vi "frontEnd.vi"() -> ()   [LabVIEW 2016]
uses:
  <userlib>/atmcd64d.llb/Error Code Enum typedef.ctl
  <userlib>/atmcd64d.llb/Shutter_mode typedef.ctl
  <userlib>/atmcd64d.llb/Shutter_type typedef.ctl
  <userlib>/atmcd64d.llb/FanMode_mode typedef.ctl
  <userlib>/atmcd64d.llb/ReadMode_mode typedef.ctl
  <userlib>/atmcd64d.llb/HSSpeed_type typedef.ctl
  <userlib>/atmcd64d.llb/AcquisitionMode_mode typedef.ctl
  <vilib>/Utility/miscctls.llb/LVStringsAndValuesArrayTypeDef_U16.ctl
  <vilib>/Utility/config.llb/Read Key (I32).vi
  <vilib>/Utility/config.llb/Read Key (Double).vi
  <vilib>/Instr/_visa.llb/VISA Configure Serial Port (Instr).vi
  <vilib>/Utility/config.llb/Read Key (String).vi
  <vilib>/Utility/config.llb/Write Key (String).vi
  <vilib>/Utility/config.llb/NI_LVConfig.lvlib
  lib/SSClassic_USBCamera_SDK.dll
panel:
  in  "String":string
  in  "Exposure Time:":dbl(slide) scale=1.0..100.0
  out "ET Labelµ":dbl format="%#_3g"
  out "new picture":picture
  in  "Red Gain":i32(slide)=20 scale=1.0..64.0
  in  "Green Gain":i32(slide)=16 scale=1.0..64.0
  in  "Blue Gain":i32(slide)=17 scale=1.0..64.0
  in  "Gain?":bool
  in  "gamma":i32=10 min=1 max=20
  in  "contrast":i32=50 min=0 max=100
  in  "bright":i32=50 min=0 max=100
  in  "sharp":i32 min=0 max=3
  out "ModuleNo:":string
  out "SerialNo:":string
  out "OK to run":bool
  in  "OM":bool
  out "relative seconds 2":dbl format="%_19f"
  out "relative seconds":dbl format="%_19f"
  out "Moving":bool
  in  "Go Origin":bool caption="Origin Return"
  in  "Set Origin":bool
  in  "Stage Position":string
  out "Cooler":bool
  out "Constructing data":u8(slide) scale=0.0..256.0
  in  "Go back after scan":bool=TRUE
  in  "Scan Step (um)":dbl
  in  "Step length (um)":dbl=100.0
  in  "go left Button":bool
  in  "go right Button":bool
  out "Y":dbl
  out "X":dbl
  in  "Scan again":bool
  in  "path":path
  in  "Bandwidth":dbl
  in  "Wavelength":i32(slide) scale=316.10943603515625..1105.4000244140625
  out "Waveform Graph":i32[](graph)
  out "Right Graph":i32[][](graph) caption="Object Image"
  out "recovering temperature":bool
  out "Left Graph":i32[][](graph) caption="On Sensor Image"
  out "Numeric 2":i32
  out "temp. status 2":T1
  out "model":string
  out "DLL error code from ini":u32
  in  "Save File":bool
  in  "Shut Down":bool
  in  "Scan Abort":bool
  out "Current \nScan Frame":dbl
  out "Total \nScan Frame":dbl
  in  "Scan Start":bool
  in  "Scan Length (mm)":dbl=25.0
  in  "Shutter Control":T2
  in  "Exposure Time (s)":sgl=0.01 step=0.001 format="%.4f"
  in  "Take shot":bool
  in  "VSS (s)":u16(ring) items=["0.300000", "0.500000", "0.900000", "1.700000", "3.300000"]
  in  "HSS (MHz)":i32(ring) items=["3", "1"]
  in  "Live View":bool
  out "Status":T1
  out "Temp":dbl
  in  "Set Temp.":dbl=20.0
  in  "Init File":path=path "C:/Users/Administrator/Desktop/micro.ini"
  # "Image Settigns"
  # "Stage Control"
  # "Scan"
  # "Save and Restart"
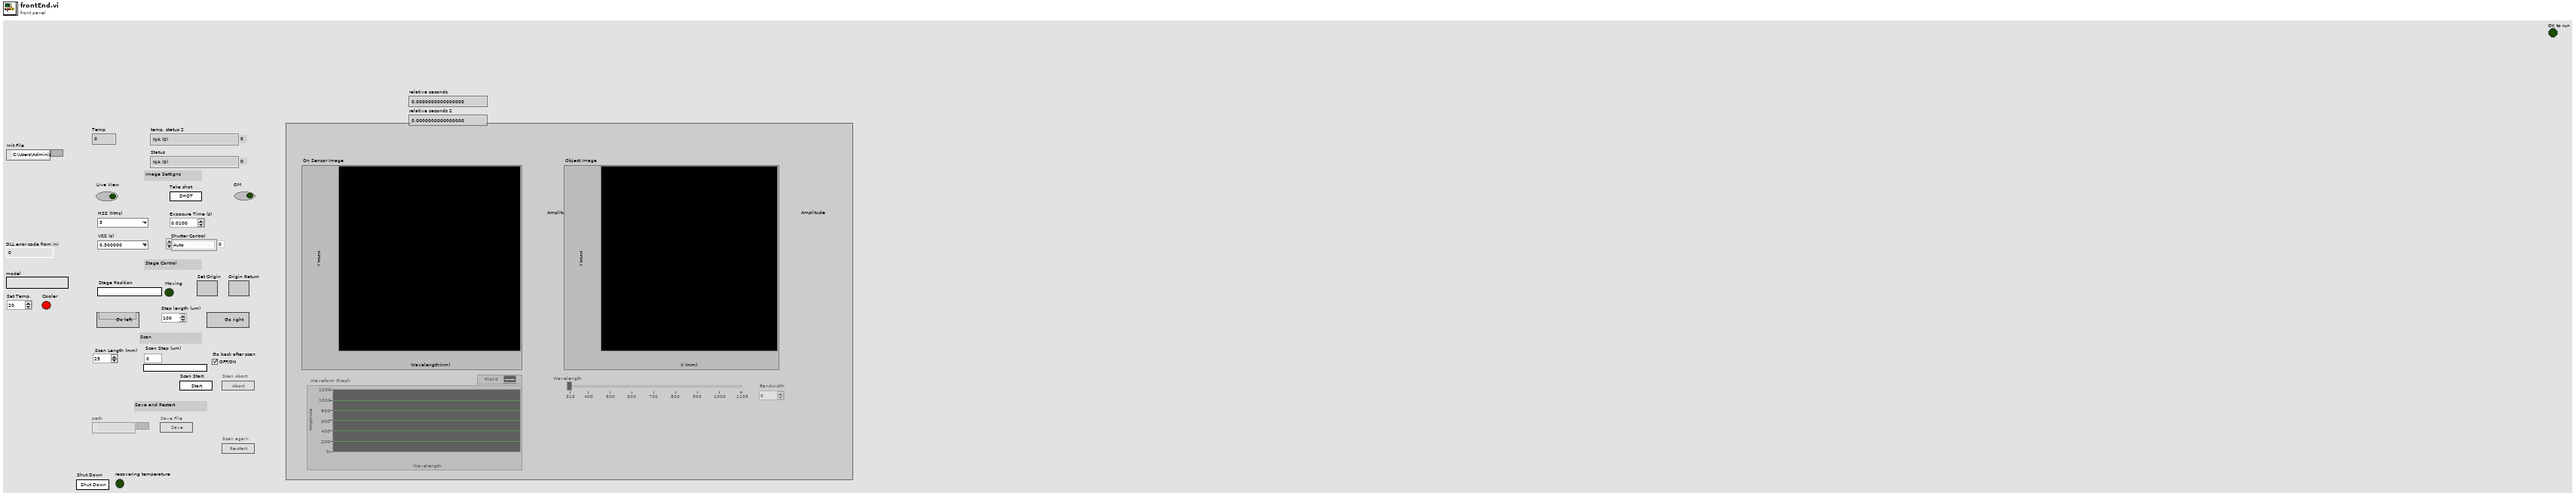
[diagram p1: front panel]
types:
  T1 = typedef "Error Code Enum typedef.ctl" = enum32{"N/A (0)", "DRV_ERROR_CODES", "DRV_SUCCESS", "DRV_VXDNOTINSTALLED", "DRV_ERROR_SCAN", "DRV_ERROR_CHECK_SUM", "DRV_ERROR_FILELOAD", "DRV_UNKNOWN_FUNC", "DRV_ERROR_VXD_INIT", "DRV_ERROR_ADDRESS", "DRV_ERROR_PAGELOCK", "DRV_ERROR_PAGEUNLOCK", "DRV_ERROR_BOARDTEST", "DRV_ERROR_ACK", "DRV_ERROR_UP_FIFO", "DRV_ERROR_PATTERN", "N/A (16)", "DRV_ACQUISITION_ERRORS", "DRV_ACQ_BUFFER", "DRV_ACQ_DOWNFIFO_FULL", "DRV_PROC_UNKONWN_INSTRUCTION", "DRV_ILLEGAL_OP_CODE", "DRV_KINETIC_TIME_NOT_MET", "DRV_ACCUM_TIME_NOT_MET", "DRV_NO_NEW_DATA", "N/A (25)", "DRV_SPOOLERROR", "N/A (27)", "N/A (28)", "N/A (29)", "N/A (30)", "N/A (31)", "N/A (32)", "DRV_TEMPERATURE_CODES", "DRV_TEMPERATURE_OFF", "DRV_TEMPERATURE_NOT_STABILIZED", "DRV_TEMPERATURE_STABILIZED", "DRV_TEMPERATURE_NOT_REACHED", "DRV_TEMPERATURE_OUT_RANGE", "DRV_TEMPERATURE_NOT_SUPPORTED", "DRV_TEMPERATURE_DRIFT", "N/A (41)", "N/A (42)", "N/A (43)", "N/A (44)", "N/A (45)", "N/A (46)", "N/A (47)", "N/A (48)", "DRV_GENERAL_ERRORS", "DRV_INVALID_AUX", "DRV_COF_NOTLOADED", "DRV_FPGAPROG", "DRV_FLEXERROR", "DRV_GPIBERROR", "N/A (55)", "N/A (56)", "N/A (57)", "N/A (58)", "N/A (59)", "N/A (60)", "N/A (61)", "N/A (62)", "N/A (63)", "DRV_DATATYPE", "DRV_DRIVER_ERRORS", "DRV_P1INVALID", "DRV_P2INVALID", "DRV_P3INVALID", "DRV_P4INVALID", "DRV_INIERROR", "DRV_COFERROR", "DRV_ACQUIRING", "DRV_IDLE", "DRV_TEMPCYCLE", "DRV_NOT_INITIALIZED", "DRV_P5INVALID", "DRV_P6INVALID", "DRV_INVALID_MODE", "DRV_INVALID_FILTER", "DRV_I2CERRORS", "DRV_I2CDEVNOTFOUND", "DRV_I2CTIMEOUT", "DRV_P7INVALID", "N/A (84)", "N/A (85)", "N/A (86)", "N/A (87)", "N/A (88)", "N/A (89)", "DRV_IOCERROR", "DRV_VRMVERSIONERROR"}
  T2 = typedef "Shutter_mode typedef.ctl" = enum16{"Auto", "Open", "Close", "N/A (3)", "Open FVB Series", "Open Any Series"}
  T3 = cluster{"Distance":i32, "Focal length":i32, "Y Range":i32}
  T4 = enum16{"open", "replace", "create", "open or create", "replace or create", "replace or create with confirmation"}
  T5 = typedef "FanMode_mode typedef.ctl" = enum16{"fan on full", "fan on low", "fan off"}
  T6 = typedef "Shutter_type typedef.ctl" = enum16{"TTL Low", "TTL High"}
  T7 = typedef "LVStringsAndValuesArrayTypeDef_U16.ctl" = cluster{"String":string, "Value":u16}[]
  T8 = typedef "AcquisitionMode_mode typedef.ctl" = enum16{"Reserved (0)", "Single Scan", "Accumulate", "Kinetics", "Fast Kinetics", "Run Till Abort", "Reserved (6)", "Reserved (7)", "Reserved (8)", "Time Delayed Integration"}
  T9 = typedef "ReadMode_mode typedef.ctl" = enum16{"Full Vertical Binning", "Multi-Track", "Random-Track", "Single-Track", "Image"}
  T10 = typedef "HSSpeed_type typedef.ctl" = enum16{"EM Amp", "Conventional Amp"}
  T11 = enum8{"Enabled", "Disabled", "Disabled and Grayed Out"}
  T12 = typedef "NI_LVConfig.lvlib/Config Data RefNum.ctl" = refnum<k1>
  T13 = typedef "imagedata.ctl" = cluster{"image type":i32, "image depth":i32, "image":u8[], "mask":u8[], "colors":u32[], "Rectangle":cluster{"left":i16, "top":i16, "right":i16, "bottom":i16}}
  T14 = typedef "LVPoint32TypeDef.ctl" = cluster{"Horizontal":i32, "Vertical":i32}
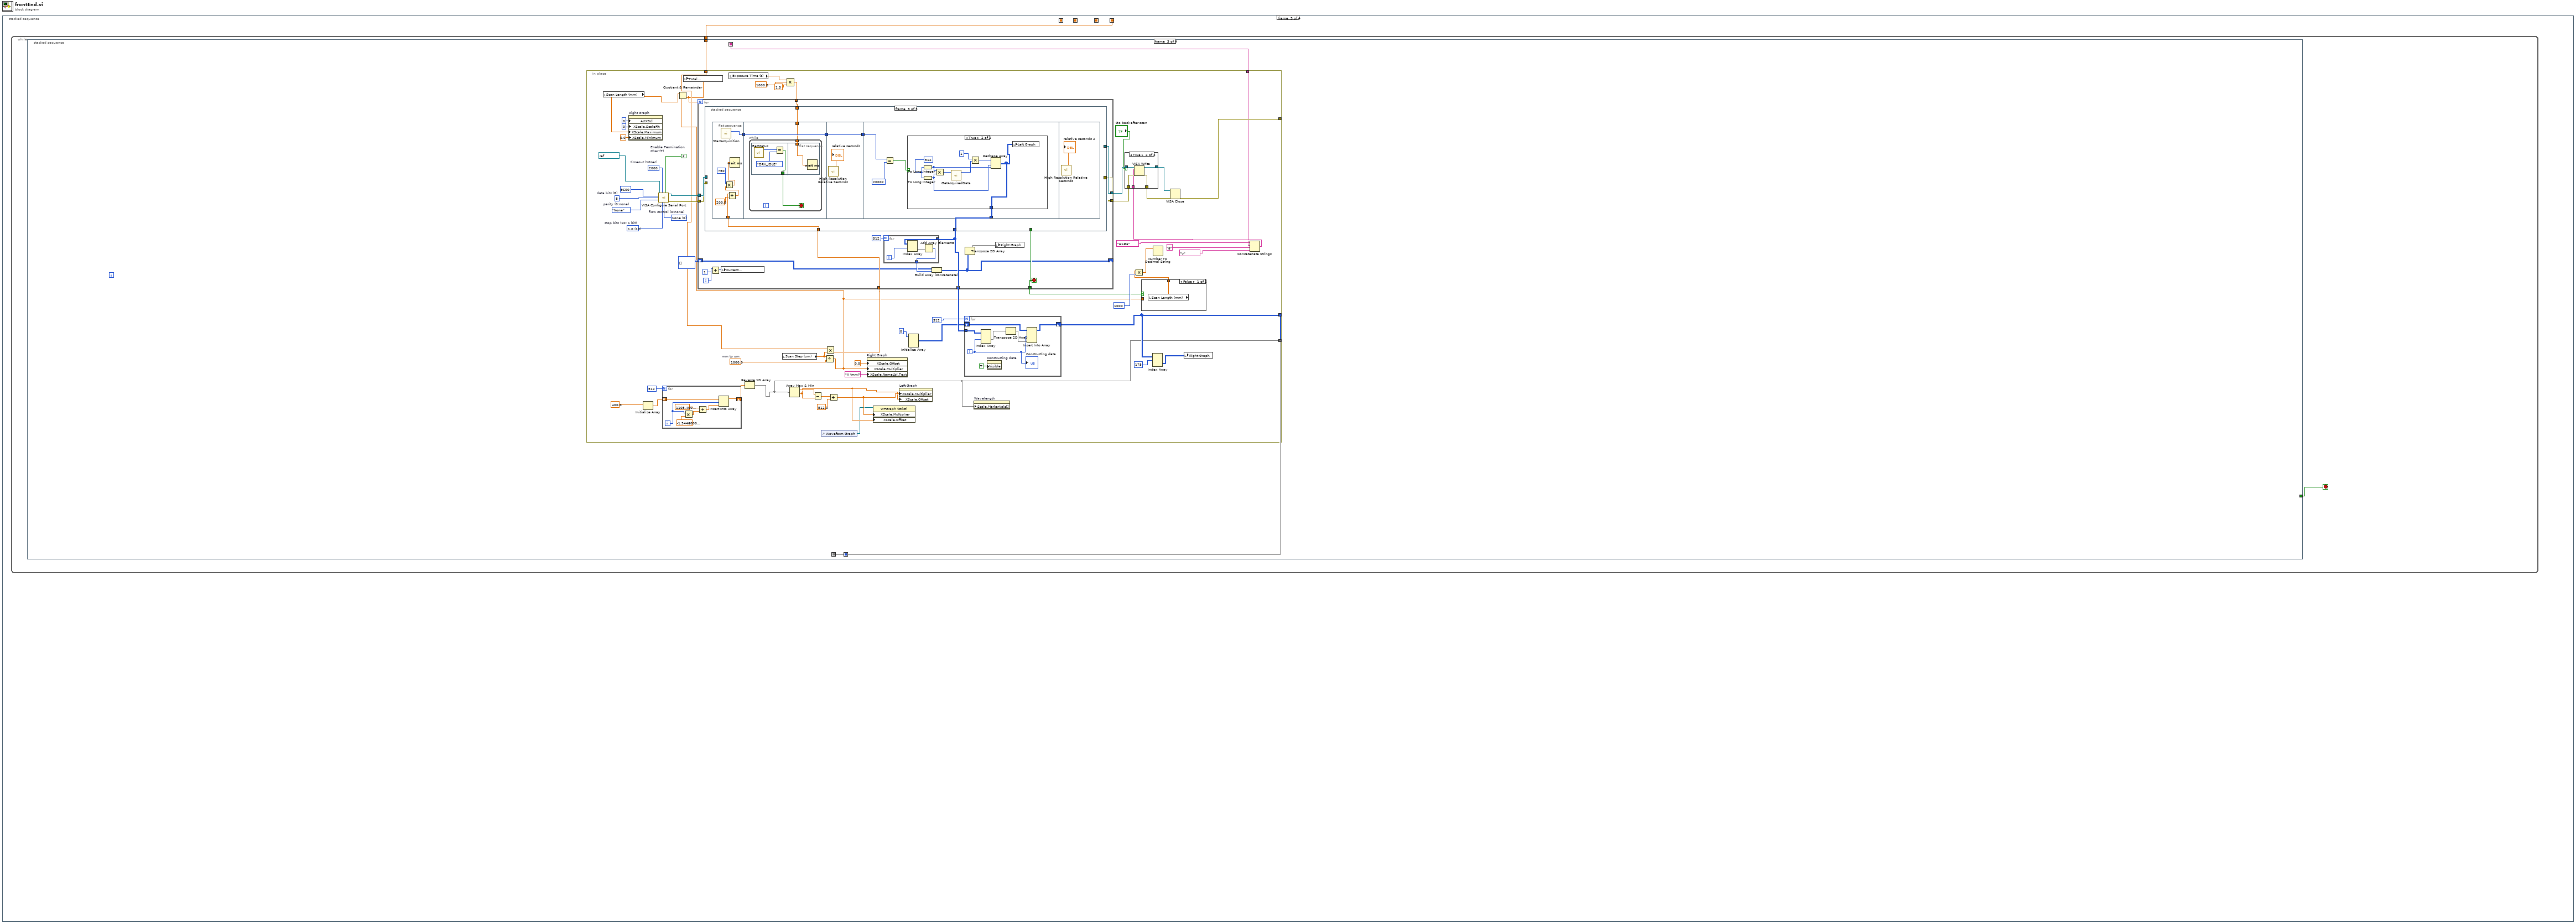
[diagram p0: block diagram]
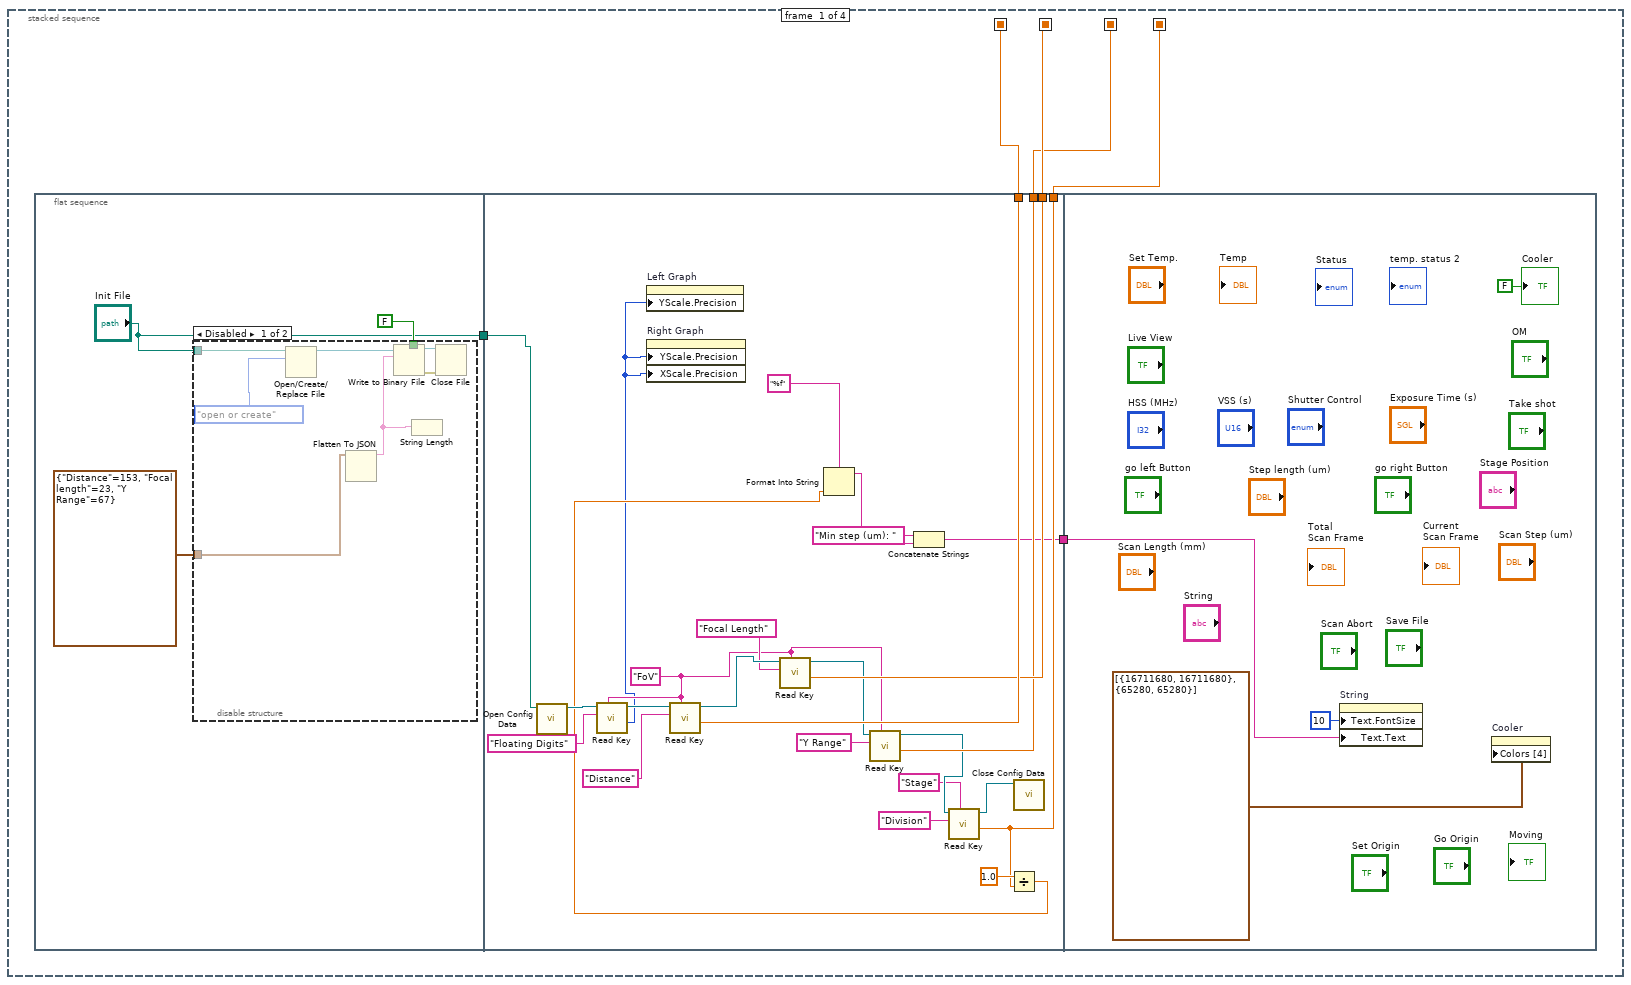
[diagram p2: hidden frame]
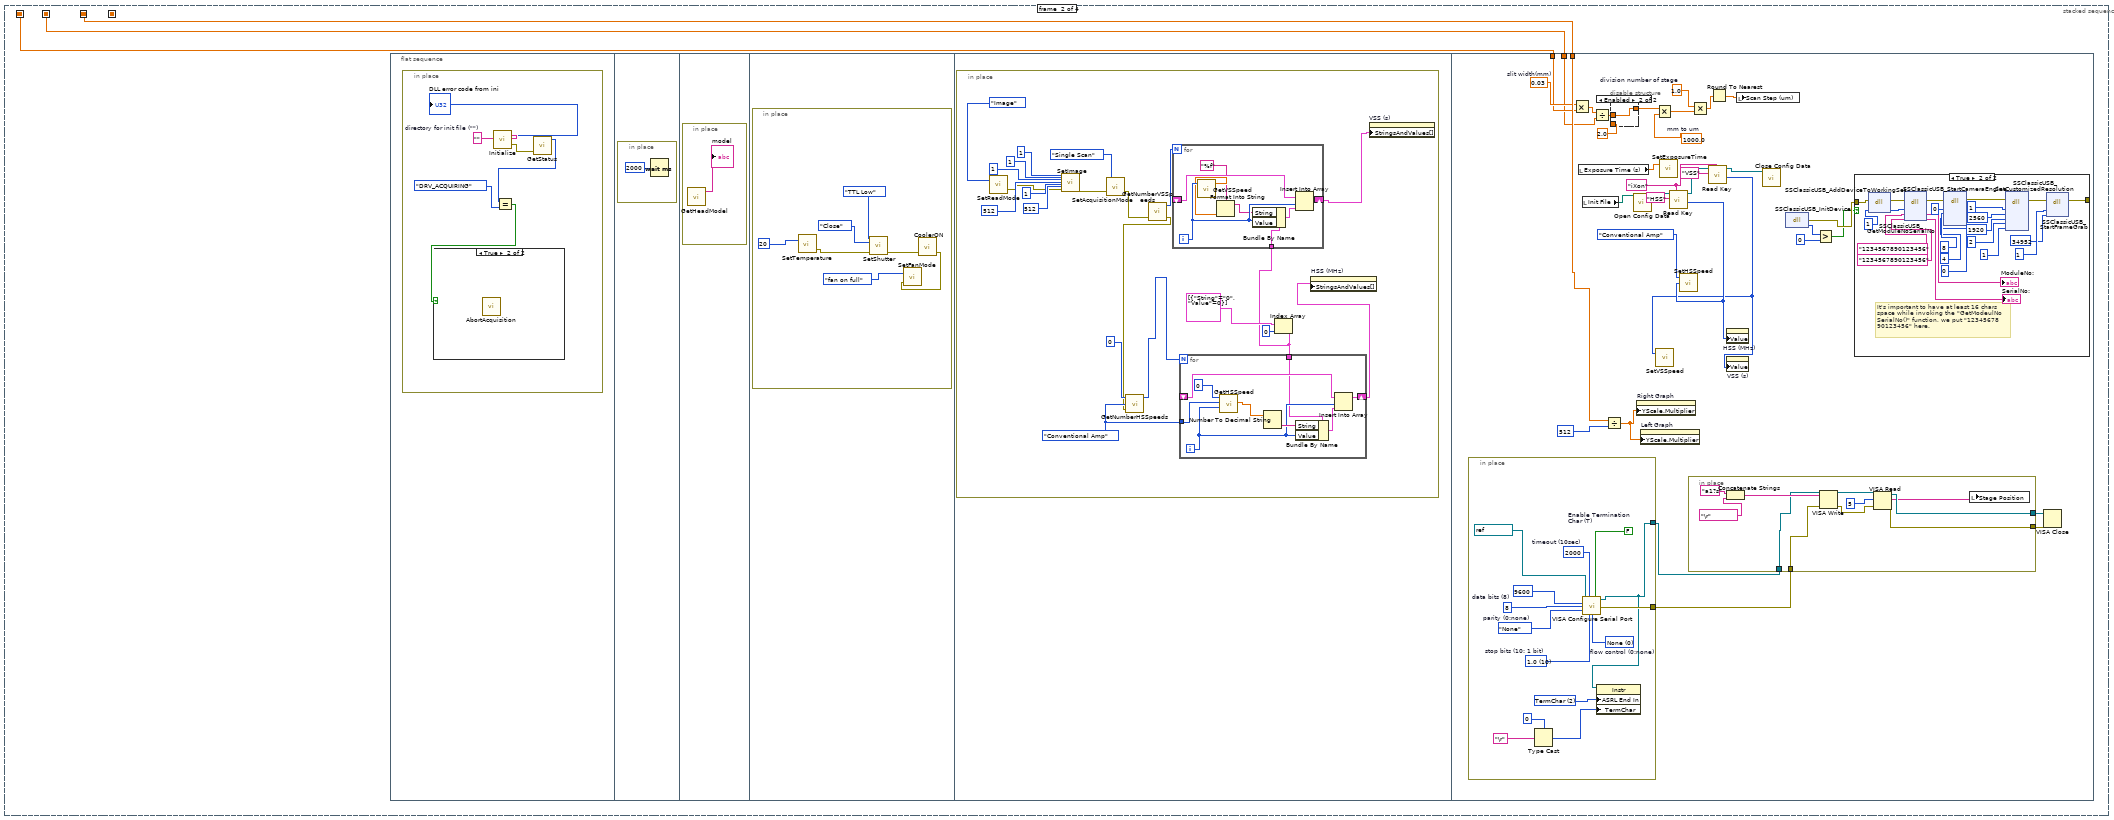
[diagram p4: hidden frame]
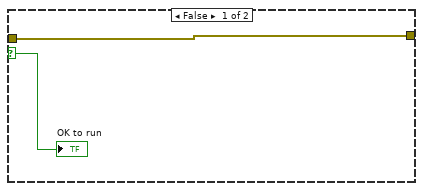
[diagram p6: hidden frame]
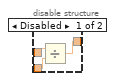
[diagram p7: hidden frame]
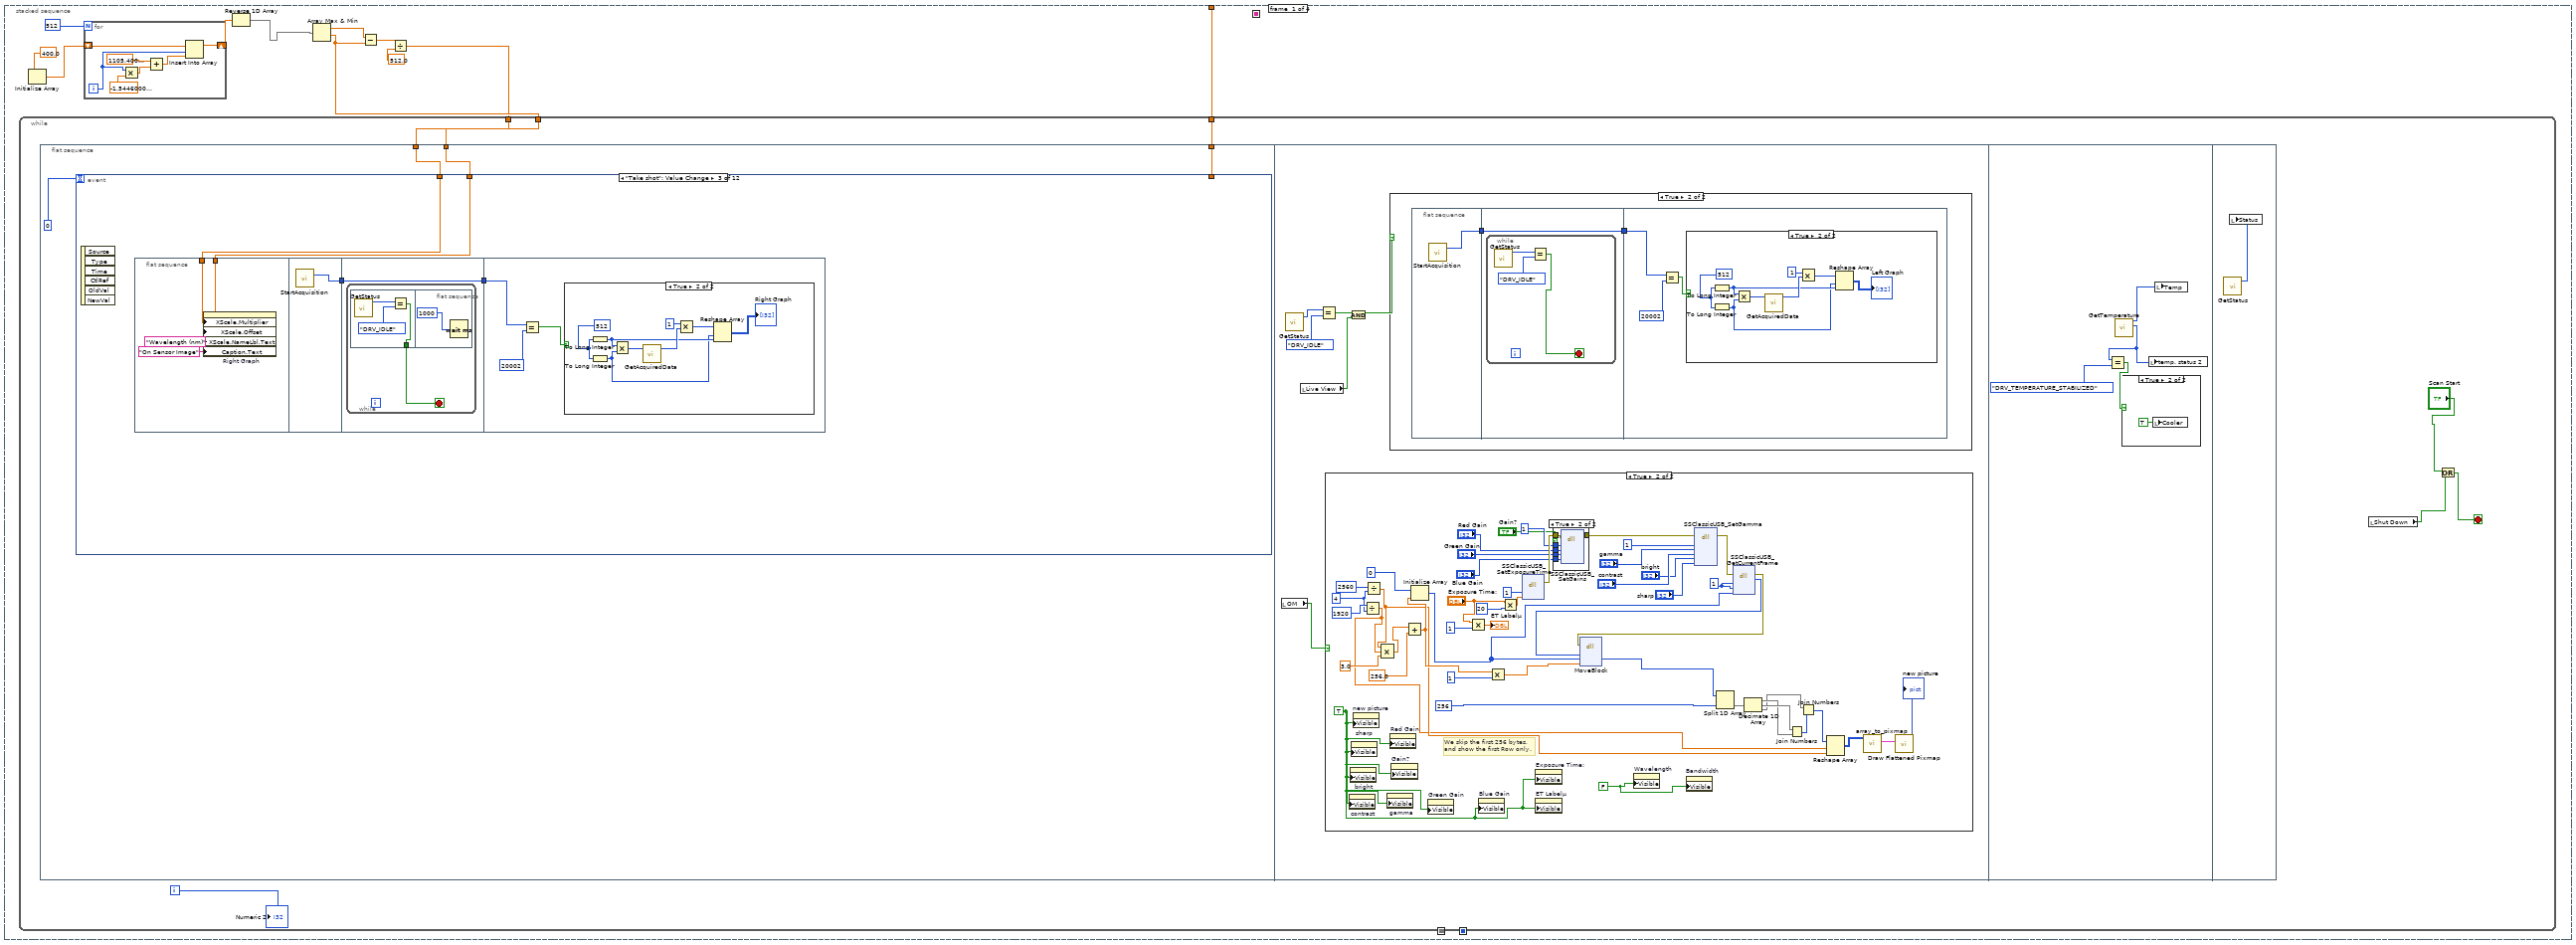
[diagram p8: hidden frame]
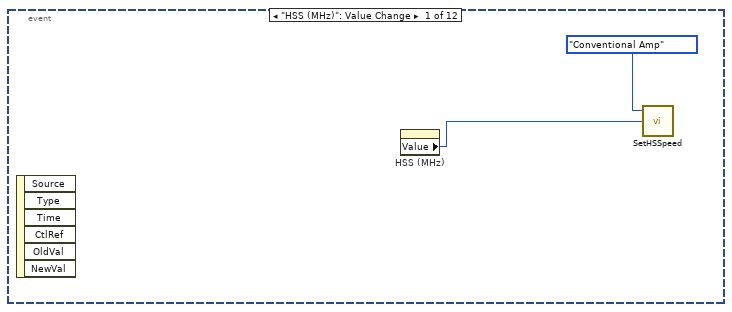
[diagram p9: hidden frame]
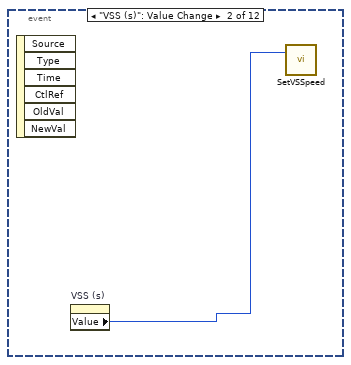
[diagram p10: hidden frame]
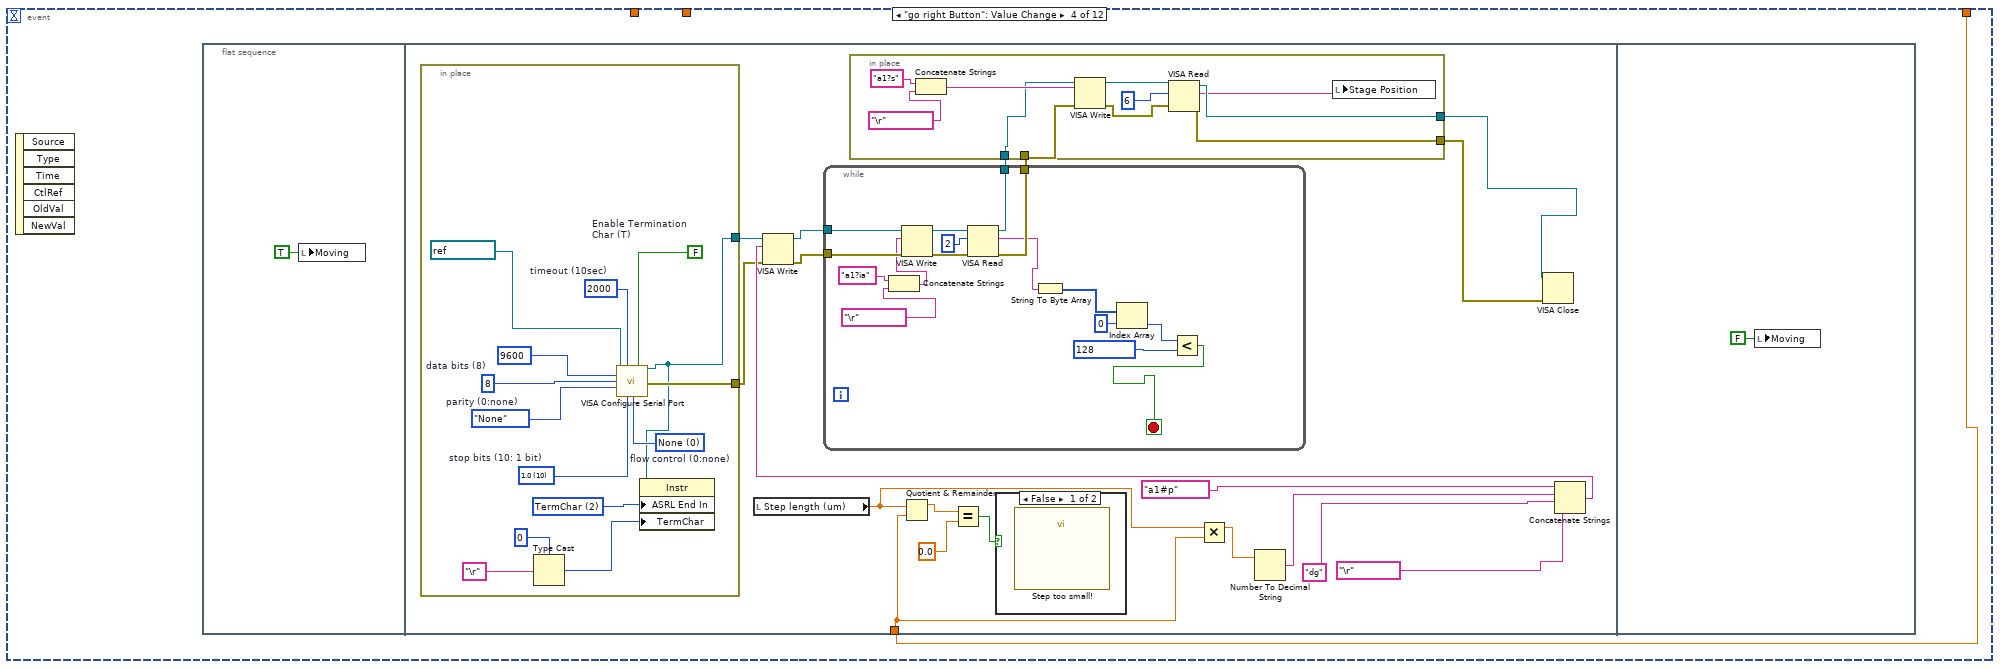
[diagram p12: hidden frame]
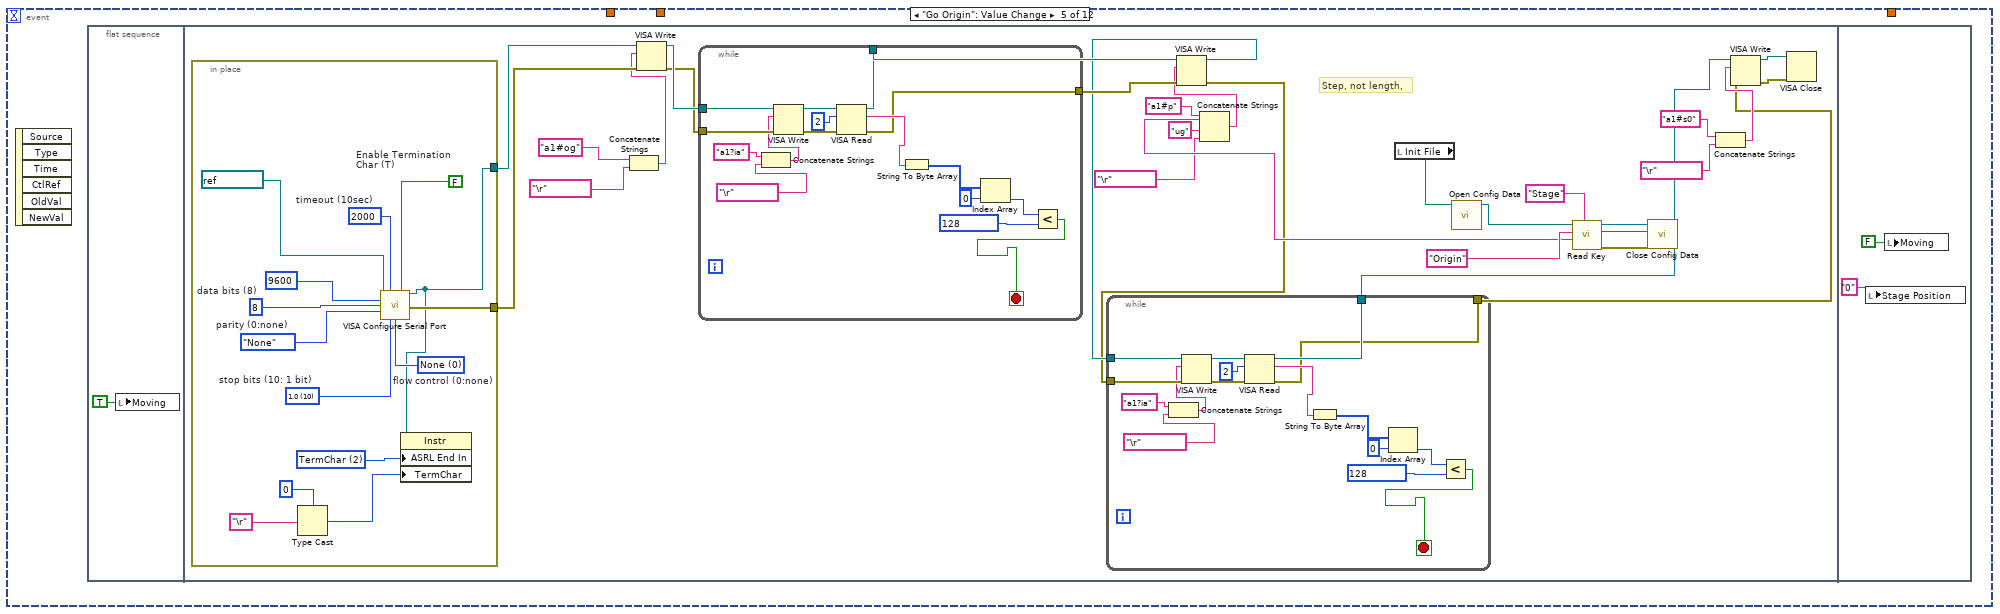
[diagram p14: hidden frame]
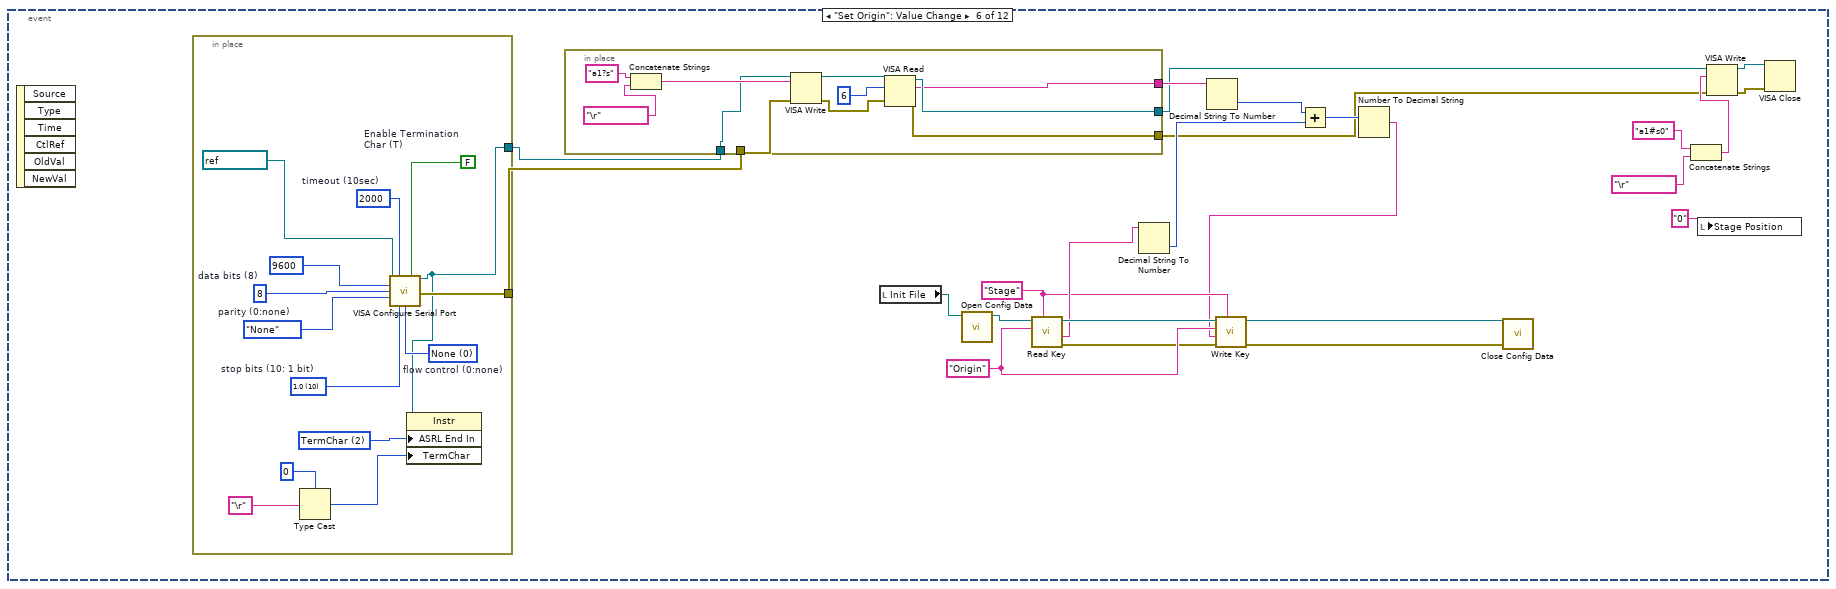
[diagram p15: hidden frame]
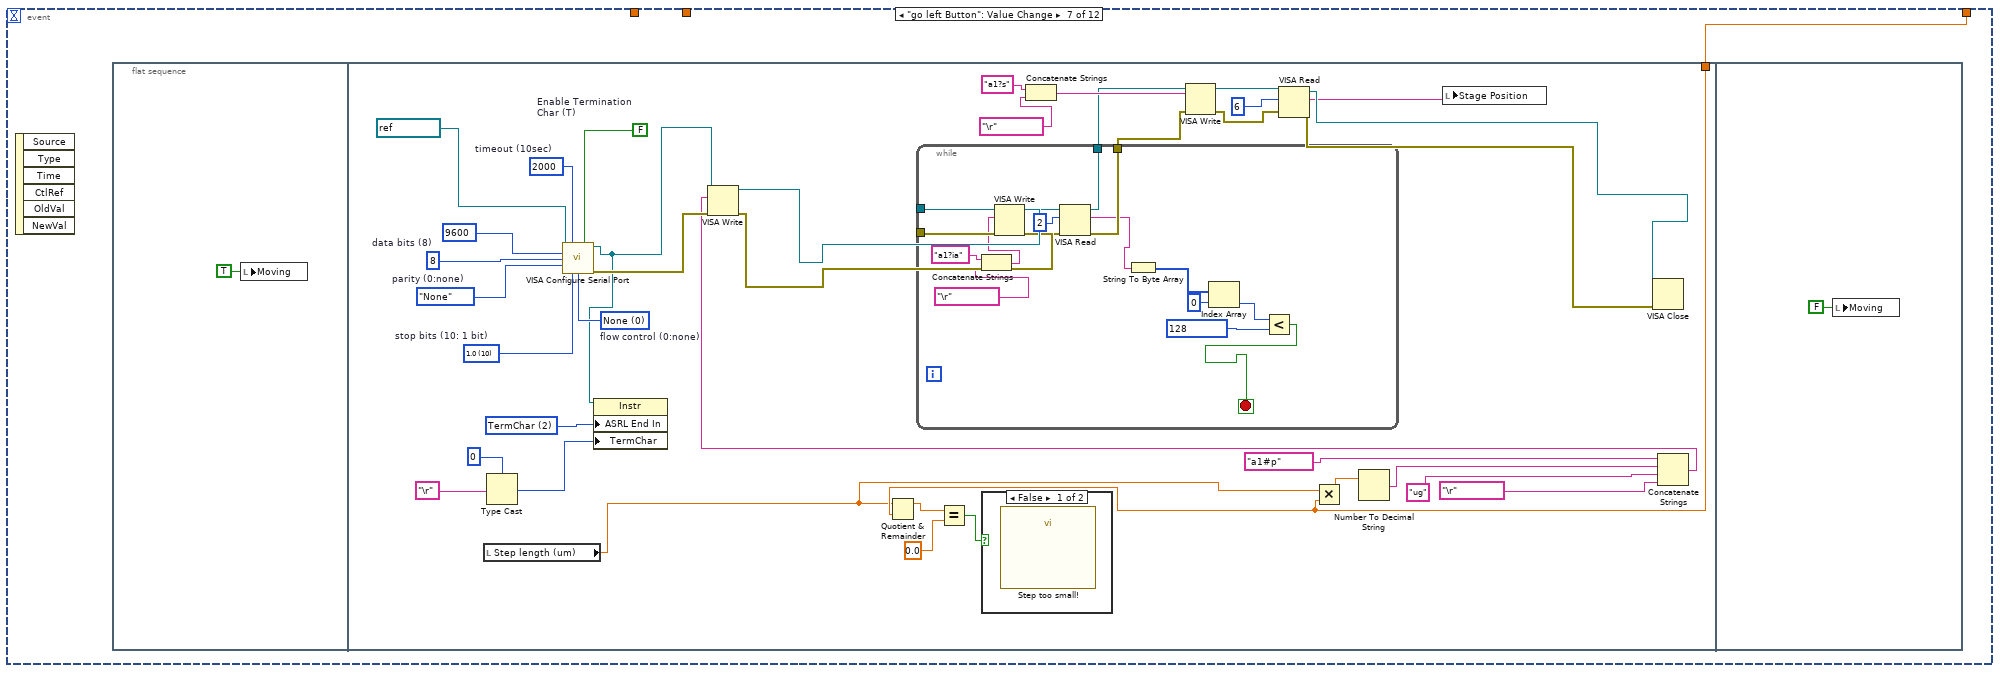
[diagram p16: hidden frame]
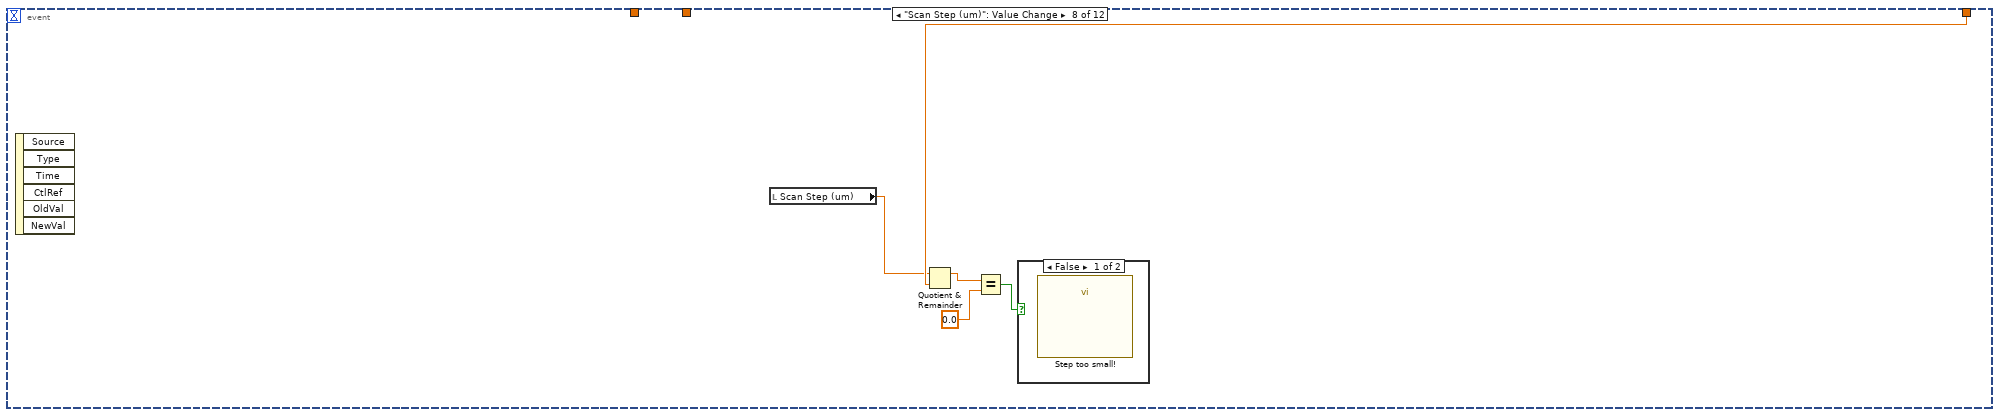
[diagram p18: hidden frame]
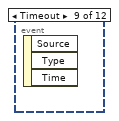
[diagram p20: hidden frame]
diagram:
  n1 = stacked-sequence {
    seq-local: [w5 _ _ _] -> [_ w48 _ _]
    seq-local: [w4 _ _ _] -> [_ w47 _ _]
    seq-local: [w3 _ _ _] -> [_ w49 _ _]
    seq-local: [w2 _ _ _] -> [_ _ w191 _]
    frame #0 {
      n2 = flat-sequence {
        tunnel: ["Init File"] -> w6
        tunnel: w6 -> [w42]
        tunnel: [w39] -> w5
        tunnel: [w36] -> w4
        tunnel: [w33] -> w3
        tunnel: [w27] -> w2
        tunnel: [w22] -> w1
        tunnel: w1 -> [w43]
        frame #0 {
          n3 = disable-structure shown="Disabled" {
            disable-tunnel: T3 {"Distance"=153, "Focal length"=23, "Y Range"=67} -> [w14 _]
            disable-tunnel: FALSE ("prepend array or string size? (T)") -> [w13 _]
            disable-tunnel: "Init File" -> [w11 _]
            frame Disabled {
              n4 = Open/Create/Replace File(file path (use dialog)=w11, operation (0:open)=T4."open or create") -> (refnum out=w15:refnum<file>)  [unwired: 4 in, 2 out]
              n5 = Flatten To JSON(anything=w14) -> (JSON string=w10:string)  [unwired: 2 in, 1 out]
              n6 = Write to Binary File(file (use dialog)=w15, data=w10, 5:w13) -> (refnum out=w17:refnum<file>, error out=w16:errorcluster)  [unwired: 3 in, 1 out]
              n7 = String Length(string=w10) -> ()  [unwired: 1 out]
              n8 = Close File(refnum=w17, error in=w16) -> ()  [unwired: 2 out]
            }
            frame Enabled {
            }
          }
        }
        frame #1 {
          w20 = "FoV" ("section")
          n9 = call <vilib>:"Open Config Data.vi"("configuration file path"=w42) -> ("refnum"=w41:T12)  [unwired: 8 in, 2 out]
          n10 = call-poly <vilib>:"Read Key.vi"("section"=w20, "key"="Floating Digits", "refnum"=w41) -> ("value"=w18:i32, "refnum out"=w21:T12)  [unwired: 5 in, 2 out]
          n11 = property on="Left Graph" class="IntGraph (strict)"("YScale.Precision"=w18) -> ()  [unwired: 2 in, 2 out]
          n12 = property on="Right Graph" class="IntGraph (strict)"("YScale.Precision"=w18, "XScale.Precision"=w18) -> ()  [unwired: 2 in, 2 out]
          n13 = call-poly <vilib>:"Read Key.vi"("section"=w20, "key"="Distance", "refnum"=w21) -> ("value"=w39:dbl, "refnum out"=w38:T12)  [unwired: 5 in, 2 out]
          n14 = call-poly <vilib>:"Read Key.vi"("section"=w20, "key"="Focal Length", "refnum"=w38) -> ("value"=w36:dbl, "refnum out"=w35:T12)  [unwired: 5 in, 2 out]
          n15 = call-poly <vilib>:"Read Key.vi"("section"=w20, "key"="Y Range", "refnum"=w35) -> ("value"=w33:dbl, "refnum out"=w32:T12)  [unwired: 5 in, 2 out]
          n16 = call-poly <vilib>:"Read Key.vi"("section"="Stage", "key"="Division", "refnum"=w32) -> ("value"=w27:dbl, "refnum out"=w31:T12)  [unwired: 5 in, 2 out]
          n17 = Divide(x=1.0, y=w27) -> (x/y=w25:dbl)
          n18 = Format Into String(format string="%f", w25) -> (resulting string=w24:string)  [unwired: 2 in, 1 out]
          n19 = Concatenate Strings("Min step (um): " ("string"), w24) -> (w22:string)
          n20 = call <vilib>:"Close Config Data.vi"("refnum"=w31) -> ()  [unwired: 9 in, 2 out]
        }
        frame #2 {
          n21 = property on="String" class="Str"("Text.FontSize"=u32 10 ("Text.Font:Size"), "Text.Text"=w43) -> ()  [unwired: 2 in, 2 out]
          n22 = property on="Cooler" class="Bool (strict)"("Colors [4]"=cluster{u32, u32}[] [{16711680, 16711680}, {65280, 65280}]) -> ()  [unwired: 2 in, 2 out]
          "Cooler" <- FALSE ("Cooler")
        }
      }
    }
    frame #1 {
      n23 = flat-sequence {
        tunnel: w49 -> [w134]
        tunnel: w48 -> [w122]
        tunnel: w47 -> [w121]
        frame #0 {
          n24 = in-place {
            w55 = ""  # directory for init file ("")
            n25 = call <userlib>:"Initialize.vi"("directory (\"\")"=w55) -> ("error out"=w53:errorcluster, "DLL error code"=→"DLL error code from ini":u32)  [unwired: 1 in]
            n26 = call <userlib>:"GetStatus.vi"("error in (no error)"=w53) -> ("status"=w52:T1)  [unwired: 2 in, 2 out]
            n27 = Equal?(x=w52, y=Error_Code_Enum_typedef."DRV_ACQUIRING" ("status")) -> (x = y?=w50:bool)
            n28 = case shown="True" w50 {
              frame False {
              }
              frame True {
                n29 = call <userlib>:"AbortAcquisition.vi"() -> ()  [unwired: 2 in, 2 out]
              }
            }
          }
        }
        frame #1 {
          n30 = in-place {
            n31 = Wait (ms)(milliseconds to wait=u32 2000) -> ()  [unwired: 1 out]
          }
        }
        frame #2 {
          n32 = in-place {
            n33 = call <userlib>:"GetHeadModel.vi"() -> ("model"=→"model":string)  [unwired: 3 in, 2 out]
          }
        }
        frame #3 {
          n34 = in-place {
            n35 = call <userlib>:"SetTemperature.vi"("temperature"=20) -> ("error out"=w61:errorcluster)  [unwired: 1 in, 1 out]
            n36 = call <userlib>:"SetShutter.vi"("type"=Shutter_type_typedef."TTL Low", "mode"=Shutter_mode_typedef."Close", "error in (no error)"=w61) -> ("error out"=w62:errorcluster)  [unwired: 11 in, 1 out]
            n37 = call <userlib>:"CoolerON.vi"("error in (no error)"=w62) -> ("error out"=w59:errorcluster)  [unwired: 1 in, 1 out]
            n38 = call <userlib>:"SetFanMode.vi"("error in (no error)"=w59, "mode"=FanMode_mode_typedef."fan on full") -> ()  [unwired: 2 out]
          }
        }
        frame #4 {
          n39 = in-place {
            w75 = HSSpeed_type_typedef."Conventional Amp" ("type")
            n40 = call <userlib>:"SetReadMode.vi"("mode"=ReadMode_mode_typedef."Image") -> ("error out"=w78:errorcluster)  [unwired: 1 in, 1 out]
            n41 = call <userlib>:"SetImage.vi"("hbin"=1, "vbin"=1, "hstart"=1, "hend"=512, "vstart"=1, "vend"=512, "error in (no error)"=w78) -> ("error out"=w72:errorcluster)  [unwired: 19 in, 1 out]
            n42 = call <userlib>:"SetAcquisitionMode.vi"("error in (no error)"=w72, "mode"=AcquisitionMode_mode_typedef."Single Scan") -> ("error out"=w71:errorcluster)  [unwired: 1 out]
            n43 = call <userlib>:"GetNumberVSSpeeds.vi"("error in (no error)"=w71) -> ("error out"=w73:errorcluster, "number"=w77:i32)  [unwired: 2 in, 1 out]
            n44 = call <userlib>:"GetNumberHSSpeeds.vi"("error in (no error)"=w73, "type"=w75, "channel"=0) -> ("number"=w74:i32)  [unwired: 2 out]
            n45 = Index Array(array=T7 [{"String"="0", "Value"=0}] ("Strings And Values []"), index=0) -> (element=w67:cluster{"String":string, "Value":u16})
            n46 = for {
              N: w77 -> [_]
              tunnel: w67 -> [w102]
              shift-right: [w99] -> w66
              shift-left: _ -> [w98]
              i -> [w100]
              n47 = call <userlib>:"GetVSSpeed.vi"("index"=w100) -> ("speed"=w96:sgl)  [unwired: 2 in, 2 out]
              n48 = Format Into String(format string="%f", w96) -> (resulting string=w97:string)  [unwired: 2 in, 1 out]
              n49 = Bundle By Name(cluster=w102, "String"=w97, "Value"=w100) -> (w101:cluster{"String":string, "Value":u16})
              n50 = Insert Into Array(array=w98, index=w100, new element=w101) -> (w99:cluster{"String":string, "Value":u16}[])
            }
            n51 = for {
              N: w74 -> [_]
              tunnel: w75 -> [w93]
              shift-right: [w88] -> w65
              shift-left: _ -> [w87]
              tunnel: w67 -> [w86]
              i -> [w89]
              n52 = call <userlib>:"GetHSSpeed.vi"("index"=w89, "type"=w93, "channel"=0) -> ("speed"=w92:sgl)  [unwired: 2 in, 2 out]
              n53 = Number To Decimal String(number=w92) -> (decimal integer string=w91:string)  [unwired: 1 in]
              n54 = Bundle By Name(cluster=w86, "String"=w91, "Value"=w89) -> (w90:cluster{"String":string, "Value":u16})
              n55 = Insert Into Array(array=w87, index=w89, new element=w90) -> (w88:cluster{"String":string, "Value":u16}[])
            }
            n56 = property on="HSS (MHz)" class="Ring (strict)"("StringsAndValues[]"=w65) -> ()  [unwired: 2 in, 2 out]
            n57 = property on="VSS (s)" class="Ring (strict)"("StringsAndValues[]"=w66) -> ()  [unwired: 2 in, 2 out]
          }
        }
        frame #5 {
          w114 = "iXon" ("section")
          w128 = 1.0  # division number of stage
          w123 = 1000.0  # mm to um
          w131 = 0.03  # slit width(mm)
          n58 = in-place {
            in-place-border: [w162] -> w107
            in-place-border: [w167] -> w110
            w163 = u16 2 items=["None", "Last Bit", "TermChar"] ("Serial Settings:End Mode for Reads")
            w169 = u16 0 items=["None", "XON/XOFF", "RTS/CTS", "XON/XOFF & RTS/CTS", "DTR/DSR", "XON/XOFF & DTR/DSR"]  # flow control (0:none)
            w170 = u16 10 items=["1.0"=10, "1.5"=15, "2.0"=20]  # stop bits (10: 1 bit)
            w171 = FALSE  # Enable Termination Char (T)
            w172 = u32 2000  # timeout (10sec)
            w173 = enum16{"None", "Odd", "Even", "Mark", "Space"}."None"  # parity (0:none)
            w174 = u16 8  # data bits (8)
            n59 = Type Cast(type=u8 0, x="\r") -> (*(type *) &x=w165:u8)
            n60 = call-poly "VISA Configure Serial Port"("VISA resource name"=refnum<visa-resource-name> "COM4", "timeout (10sec)"=w172, "Enable Termination\nChar (T)"=w171, "baud rate (9600)"=u32 9600, "data bits (8)"=w174, "parity (0:none)"=w173, "stop bits (10: 1 bit)"=w170, "flow control (0:none)"=w169) -> ("VISA resource name out"=w162:refnum<visa-resource-name>, "error out"=w167:errorcluster)  [unwired: 6 in]
            n61 = property class="Instr"(reference=w162, "ASRL End In"=w163, "TermChar"=w165) -> ()  [unwired: 1 in, 2 out]
          }
          n62 = Multiply(x=w131, y=w122) -> (x*y=w130:dbl)
          n63 = local read "Exposure Time (s)"() -> (w135:sgl)
          n64 = local read "Init File"() -> (w119:path)
          n65 = Divide(x=w130, y=w121) -> (x/y=w127:dbl)
          n66 = Divide(x=w134, y=512) -> (x/y=w132:dbl)
          n67 = disable-structure shown="Enabled" {
            disable-tunnel: w127 -> [w189 w190]
            disable-tunnel: 2.0 ("y") -> [w188 _]
            disable-tunnel: [w187 w190] -> w125
            frame Disabled {
              n68 = Divide(x=w189, y=w188) -> (x/y=w187:dbl)
            }
            frame Enabled {
            }
          }
          n69 = call <vilib>:"Open Config Data.vi"("configuration file path"=w119) -> ("refnum"=w118:T12)  [unwired: 8 in, 2 out]
          n70 = property on="Right Graph" class="IntGraph (strict)"("YScale.Multiplier"=w132) -> ()  [unwired: 2 in, 2 out]
          n71 = property on="Left Graph" class="IntGraph (strict)"("YScale.Multiplier"=w132) -> ()  [unwired: 2 in, 2 out]
          n72 = Multiply(x=w125, y=w123) -> (x*y=w129:dbl)
          n73 = call <userlib>:"SetExposureTime.vi"("time"=w135) -> ()  [unwired: 1 in, 2 out]
          n74 = call-poly <vilib>:"Read Key.vi"("section"=w114, "key"="HSS", "refnum"=w118) -> ("value"=w116:i32, "refnum out"=w115:T12)  [unwired: 5 in, 2 out]
          n75 = call <userlib>:"SetHSSpeed.vi"("index"=w116, "type"=HSSpeed_type_typedef."Conventional Amp") -> ()  [unwired: 2 in, 2 out]
          n76 = in-place {
            in-place-border: w107 -> [w181]
            in-place-border: w110 -> [w180]
            in-place-border: [w179] -> w109
            in-place-border: [w178] -> w108
            n77 = Concatenate Strings("a1?s" ("write buffer"), "\r" ("write buffer")) -> (w184:string)
            n78 = VISA Write(VISA resource name=w181, write buffer=w184, error in (no error)=w180) -> (VISA resource name out=w185:refnum<visa-resource-name>, error out=w176:errorcluster)  [unwired: 1 out]
            n79 = VISA Read(VISA resource name=w185, byte count=u32 5, error in (no error)=w176) -> (VISA resource name out=w178:refnum<visa-resource-name>, read buffer=w177:string, error out=w179:errorcluster)  [unwired: 1 out]
            n80 = local write "Stage Position"(w177) -> ()
          }
          n81 = Multiply(x=w128, y=w129) -> (x*y=w124:dbl)
          n82 = call-poly <vilib>:"Read Key.vi"("section"=w114, "key"="VSS", "refnum"=w115) -> ("value"=w112:i32, "refnum out"=w111:T12)  [unwired: 5 in, 2 out]
          n83 = call <userlib>:"SetVSSpeed.vi"("index"=w112) -> ()  [unwired: 1 in, 2 out]
          n84 = Round To Nearest(number=w124) -> (nearest integer value=w120:dbl)
          n85 = property on="HSS (MHz)" class="Ring (strict)"("Value"=w116) -> ()  [unwired: 2 in, 2 out]
          n86 = property on="VSS (s)" class="Ring (strict)"("Value"=w112) -> ()  [unwired: 2 in, 2 out]
          n87 = local write "Scan Step (um)"(w120) -> ()
          n88 = call <vilib>:"Close Config Data.vi"("refnum"=w111) -> ()  [unwired: 9 in, 2 out]
          n89 = dll-call lib="D:/All users/PoSheng/src/lib/SSClassic_USBCamera_SDK.dll" fn="SSClassicUSB_InitDevice" ("CCD_USBCamera_SDK.dll:CCDUSB_InitDevice")() -> (error out=w104:errorcluster, "ReturnValue"=w106:u32)  [unwired: 3 in, 1 out]
          n90 = Greater?(x=w106, y=0) -> (0:w103:bool)
          n91 = case shown="True" w103 {
            selector: w103 -> [w138 _]
            tunnel: w104 -> [w137 w161]
            tunnel: [w137 w154] -> _
            frame False {
              "OK to run" <- w138
            }
            frame True {
              # "It's important to have at least 16 chars\nspace while invoking the \"GetModeulNo\nSerialNo()\" function, we put \"12345678\n90123456\" here."
              n92 = dll-call lib="D:/All users/PoSheng/src/lib/SSClassic_USBCamera_SDK.dll" fn="SSClassicUSB_AddDeviceToWorkingSet" ("CCD_USBCamera_SDK.dll:CCDUSB_AddDeviceToWorkingSet")(error in=w161, "Arg1"=1) -> (error out=w160:errorcluster, "Arg1"=w158:i32)  [unwired: 3 in, 1 out]
              n93 = dll-call lib="D:/All users/PoSheng/src/lib/SSClassic_USBCamera_SDK.dll" fn="SSClassicUSB_GetModuleNoSerialNo" ("CCD_USBCamera_SDK.dll:CCDUSB_GetModuleNoSerialNo")(error in=w160, "Arg1"=w158, "Arg2"="1234567890123456", "Arg3"="1234567890123456") -> (error out=w156:errorcluster, "Arg2"=→"ModuleNo:":string, "Arg3"=→"SerialNo:":string)  [unwired: 4 in, 1 out]
              n94 = dll-call lib="D:/All users/PoSheng/src/lib/SSClassic_USBCamera_SDK.dll" fn="SSClassicUSB_StartCameraEngine" ("CCD_USBCamera_SDK.dll:CCDUSB_StartCameraEngine")(error in=w156, "Arg1"=0, "Arg2"=8, "Arg3"=4, "Arg4"=0) -> (error out=w149:errorcluster)  [unwired: 7 in, 1 out]
              n95 = dll-call lib="D:/All users/PoSheng/src/lib/SSClassic_USBCamera_SDK.dll" fn="SSClassicUSB_SetCustomizedResolution" ("BUF_USBCamera_SDK.dll:BUFUSB_SetCustomizedResolution")(error in=w149, "Arg1"=1, "Arg2"=2560, "Arg3"=1920, "Arg4"=2, "Arg5"=u32 1) -> (error out=w148:errorcluster)  [unwired: 8 in, 1 out]
              n96 = dll-call lib="D:/All users/PoSheng/src/lib/SSClassic_USBCamera_SDK.dll" fn="SSClassicUSB_StartFrameGrab" ("CCD_USBCamera_SDK.dll:CCDUSB_StartFrameGrab")(error in=w148, "Arg1"=1, "Arg2"=34952) -> (error out=w154:errorcluster)  [unwired: 5 in, 1 out]
            }
          }
          n97 = VISA Close(VISA resource name=w108, error in (no error)=w109) -> ()  [unwired: 1 out]
        }
      }
    }
    frame #2 {
      n98 = while {
        tunnel: w191 -> [w192]
        stop <- w193 stop-if-true
        n99 = stacked-sequence {
          seq-local: [_ _ w643 _] -> [_ _ _ w801]
          seq-local: [_ _ w642 _] -> [_ _ _ w802]
          seq-local: [_ w598 _ _] -> [_ _ w641 _]
          tunnel: [_ _ _ w800] -> w193
          tunnel: w192 -> [w194 _ w640 _]
          frame #0 {
            n100 = Initialize Array(sgl 400.0 ("element")) -> (w200:sgl[])  [unwired: 1 in]
            n101 = for {
              N: 512 -> [_]
              shift-right: [w210] -> w201
              shift-left: w200 -> [w211]
              i -> [w209]
              n102 = Multiply(x=w209, y=sgl -1.5446) -> (x*y=w207:sgl)
              n103 = Add(x=sgl 1105.4, y=w207) -> (x+y=w205:sgl)
              n104 = Insert Into Array(array=w211, index=w209, new element=w205) -> (w210:sgl[])
            }
            n105 = Reverse 1D Array(array=w201) -> (reversed array=w197:sgl[])
            n106 = Array Max & Min(array=w197) -> (max value=w202:sgl, min value=w196:sgl)  [unwired: 2 out]
            n107 = Subtract(x=w202, y=w196) -> (x-y=w203:sgl)
            n108 = Divide(x=w203, y=sgl 512.0) -> (x/y=w195:sgl)
            n109 = while {
              tunnel: w196 -> [w217]
              tunnel: w195 -> [w216]
              tunnel: w194 -> [w212]
              i -> [w218]
              stop <- w213 stop-if-true
              n110 = flat-sequence {
                tunnel: w217 -> [w221]
                tunnel: w216 -> [w220]
                tunnel: w212 -> [w219]
                frame #0 {
                  n111 = event shown="[2] \"Take shot\": Value Change" {
                    selector: _ -> [_ _ _ _ _ _ _ _ _ _ _ _]
                    dyn-events: _ -> [_ _ _ _ _ _ _ _ _ _ _ _]
                    timeout: 0 -> [_ _ _ _ _ _ _ _ _ _ _ _]
                    tunnel: w221 -> [_ _ w227 _ _ _ _ _ _ _ _ _]
                    tunnel: w220 -> [_ _ w226 _ _ _ _ _ _ _ _ _]
                    tunnel: w219 -> [_ _ _ w252 _ _ w443 w501 _ _ _ _]
                    event "HSS (MHz)": Value Change {
                      n112 = event-data() -> ()  [unwired: 1 in, 6 out]
                      n113 = property on="HSS (MHz)" class="Ring (strict)"() -> ("Value"=w223:i32)  [unwired: 2 in, 2 out]
                      n114 = call <userlib>:"SetHSSpeed.vi"("index"=w223, "type"=HSSpeed_type_typedef."Conventional Amp") -> ()  [unwired: 2 in, 2 out]
                    }
                    event "VSS (s)": Value Change {
                      n115 = event-data() -> ()  [unwired: 1 in, 6 out]
                      n116 = property on="VSS (s)" class="Ring (strict)"() -> ("Value"=w225:u16)  [unwired: 2 in, 2 out]
                      n117 = call <userlib>:"SetVSSpeed.vi"("index"=w225) -> ()  [unwired: 1 in, 2 out]
                    }
                    event "Take shot": Value Change {
                      n118 = event-data() -> ()  [unwired: 1 in, 6 out]
                      n119 = flat-sequence {
                        tunnel: w227 -> [w233]
                        tunnel: w226 -> [w232]
                        tunnel: [w234] -> w229
                        tunnel: w229 -> [w235]
                        tunnel: [w235] -> w228
                        tunnel: w228 -> [w243]
                        frame #0 {
                          n120 = property on="Right Graph" class="IntGraph (strict)"("XScale.Multiplier"=w232, "XScale.Offset"=w233, "XScale.NameLbl.Text"="Wavelength (nm)" ("X Scale.Name Label.Text"), "Caption.Text"="On Sensor Image" ("Label.Text")) -> ()  [unwired: 2 in, 2 out]
                        }
                        frame #1 {
                          n121 = call <userlib>:"StartAcquisition.vi"() -> ("DLL error code"=w234:u32)  [unwired: 2 in, 1 out]
                        }
                        frame #2 {
                          n122 = while {
                            stop <- w236 stop-if-true
                            n123 = flat-sequence {
                              tunnel: [w237] -> w236
                              frame #0 {
                                n124 = call <userlib>:"GetStatus.vi"() -> ("status"=w238:T1)  [unwired: 3 in, 2 out]
                                n125 = Equal?(x=w238, y=Error_Code_Enum_typedef."DRV_IDLE" ("status")) -> (x = y?=w237:bool)
                              }
                              frame #1 {
                                n126 = Wait (ms)(milliseconds to wait=u32 1000) -> ()  [unwired: 1 out]
                              }
                            }
                          }
                        }
                        frame #3 {
                          n127 = Equal?(x=w243, y=u32 20002) -> (x = y?=w241:bool)
                          n128 = case shown="True" w241 {
                            frame False {
                            }
                            frame True {
                              w245 = 512
                              n129 = To Long Integer(number=w245) -> (32bit integer=w247:i32)
                              n130 = To Long Integer(number=w245) -> (32bit integer=w246:i32)
                              n131 = Multiply(x=w247, y=w246) -> (x*y=w251:i32)
                              n132 = call <userlib>:"GetAcquiredData.vi"("size"=w251) -> ("array"=w249:i32[])  [unwired: 2 in, 2 out]
                              n133 = Multiply(x=1, y=w249) -> (x*y=w248:i32[])
                              n134 = Reshape Array(w248, w246, w247) -> (→"Right Graph":i32[][])
                            }
                          }
                        }
                      }
                    }
                    event "go right Button": Value Change {
                      n135 = event-data() -> ()  [unwired: 1 in, 6 out]
                      n136 = flat-sequence {
                        tunnel: w252 -> [w258]
                        frame #0 {
                          n137 = local write "Moving"(TRUE ("Moving")) -> ()
                        }
                        frame #1 {
                          n138 = in-place {
                            in-place-border: [w284] -> w267
                            in-place-border: [w289] -> w266
                            w285 = u16 2 items=["None", "Last Bit", "TermChar"] ("Serial Settings:End Mode for Reads")
                            w291 = u16 0 items=["None", "XON/XOFF", "RTS/CTS", "XON/XOFF & RTS/CTS", "DTR/DSR", "XON/XOFF & DTR/DSR"]  # flow control (0:none)
                            w292 = u16 10 items=["1.0"=10, "1.5"=15, "2.0"=20]  # stop bits (10: 1 bit)
                            w293 = FALSE  # Enable Termination Char (T)
                            w294 = u32 2000  # timeout (10sec)
                            w295 = enum16{"None", "Odd", "Even", "Mark", "Space"}."None"  # parity (0:none)
                            w296 = u16 8  # data bits (8)
                            n139 = Type Cast(type=u8 0, x="\r") -> (*(type *) &x=w287:u8)
                            n140 = call-poly "VISA Configure Serial Port"("VISA resource name"=refnum<visa-resource-name> "COM4", "timeout (10sec)"=w294, "Enable Termination\nChar (T)"=w293, "baud rate (9600)"=u32 9600, "data bits (8)"=w296, "parity (0:none)"=w295, "stop bits (10: 1 bit)"=w292, "flow control (0:none)"=w291) -> ("VISA resource name out"=w284:refnum<visa-resource-name>, "error out"=w289:errorcluster)  [unwired: 6 in]
                            n141 = property class="Instr"(reference=w284, "ASRL End In"=w285, "TermChar"=w287) -> ()  [unwired: 1 in, 2 out]
                          }
                          n142 = local read "Step length (um)"() -> (w254:dbl)
                          n143 = Quotient & Remainder(x=w254, y=w258) -> (x-y*floor(x/y)=w257:dbl)  [unwired: 1 out]
                          n144 = Equal?(x=w257, y=0.0) -> (x = y?=w255:bool)
                          n145 = case shown="False" w255 {
                            frame False {
                              n146 = call "Step too small!"() -> ()  [unwired: 18 in, 2 out]
                            }
                            frame True {
                            }
                          }
                          n147 = Multiply(x=w254, y=w258) -> (x*y=w259:dbl)
                          n148 = Number To Decimal String(number=w259) -> (decimal integer string=w271:string)  [unwired: 1 in]
                          n149 = Concatenate Strings("a1#p" ("string"), w271, "dg" ("string"), "\r" ("write buffer")) -> (w272:string)
                          n150 = VISA Write(VISA resource name=w267, write buffer=w272, error in (no error)=w266) -> (VISA resource name out=w265:refnum<visa-resource-name>, error out=w264:errorcluster)  [unwired: 1 out]
                          n151 = while {
                            tunnel: w265 -> [w313]
                            tunnel: w264 -> [w312]
                            tunnel: [w305] -> w263
                            tunnel: [w304] -> w262
                            stop <- w298 stop-if-true
                            n152 = Concatenate Strings("a1?ia" ("write buffer"), "\r" ("write buffer")) -> (w309:string)
                            n153 = VISA Write(VISA resource name=w313, write buffer=w309, error in (no error)=w312) -> (VISA resource name out=w308:refnum<visa-resource-name>, error out=w307:errorcluster)  [unwired: 1 out]
                            n154 = VISA Read(VISA resource name=w308, byte count=u32 2, error in (no error)=w307) -> (VISA resource name out=w305:refnum<visa-resource-name>, read buffer=w303:string, error out=w304:errorcluster)  [unwired: 1 out]
                            n155 = String To Byte Array(string=w303) -> (unsigned byte array=w302:u8[])
                            n156 = Index Array(array=w302, index=0) -> (element=w300:u8)
                            n157 = Less?(x=w300, y=u8 128) -> (x < y?=w298:bool)
                          }
                          n158 = in-place {
                            in-place-border: w263 -> [w278]
                            in-place-border: w262 -> [w277]
                            in-place-border: [w276] -> w261
                            in-place-border: [w275] -> w260
                            n159 = Concatenate Strings("a1?s" ("write buffer"), "\r" ("write buffer")) -> (w281:string)
                            n160 = VISA Write(VISA resource name=w278, write buffer=w281, error in (no error)=w277) -> (VISA resource name out=w282:refnum<visa-resource-name>, error out=w273:errorcluster)  [unwired: 1 out]
                            n161 = VISA Read(VISA resource name=w282, byte count=u32 6, error in (no error)=w273) -> (VISA resource name out=w275:refnum<visa-resource-name>, read buffer=w274:string, error out=w276:errorcluster)  [unwired: 1 out]
                            n162 = local write "Stage Position"(w274) -> ()
                          }
                          n163 = VISA Close(VISA resource name=w260, error in (no error)=w261) -> ()  [unwired: 1 out]
                        }
                        frame #2 {
                          n164 = local write "Moving"(FALSE ("Moving")) -> ()
                        }
                      }
                    }
                    event "Go Origin": Value Change {
                      n165 = event-data() -> ()  [unwired: 1 in, 6 out]
                      n166 = flat-sequence {
                        frame #0 {
                          n167 = local write "Moving"(TRUE ("Moving")) -> ()
                        }
                        frame #1 {
                          # "Step, not length,"
                          n168 = in-place {
                            in-place-border: [w378] -> w345
                            in-place-border: [w383] -> w344
                            w379 = u16 2 items=["None", "Last Bit", "TermChar"] ("Serial Settings:End Mode for Reads")
                            w385 = u16 0 items=["None", "XON/XOFF", "RTS/CTS", "XON/XOFF & RTS/CTS", "DTR/DSR", "XON/XOFF & DTR/DSR"]  # flow control (0:none)
                            w386 = u16 10 items=["1.0"=10, "1.5"=15, "2.0"=20]  # stop bits (10: 1 bit)
                            w387 = FALSE  # Enable Termination Char (T)
                            w388 = u32 2000  # timeout (10sec)
                            w389 = enum16{"None", "Odd", "Even", "Mark", "Space"}."None"  # parity (0:none)
                            w390 = u16 8  # data bits (8)
                            n169 = Type Cast(type=u8 0, x="\r") -> (*(type *) &x=w381:u8)
                            n170 = call-poly "VISA Configure Serial Port"("VISA resource name"=refnum<visa-resource-name> "COM4", "timeout (10sec)"=w388, "Enable Termination\nChar (T)"=w387, "baud rate (9600)"=u32 9600, "data bits (8)"=w390, "parity (0:none)"=w389, "stop bits (10: 1 bit)"=w386, "flow control (0:none)"=w385) -> ("VISA resource name out"=w378:refnum<visa-resource-name>, "error out"=w383:errorcluster)  [unwired: 6 in]
                            n171 = property class="Instr"(reference=w378, "ASRL End In"=w379, "TermChar"=w381) -> ()  [unwired: 1 in, 2 out]
                          }
                          n172 = Concatenate Strings("a1#og" ("string"), "\r" ("write buffer")) -> (w341:string)
                          n173 = VISA Write(VISA resource name=w345, write buffer=w341, error in (no error)=w344) -> (VISA resource name out=w340:refnum<visa-resource-name>, error out=w339:errorcluster)  [unwired: 1 out]
                          n174 = while {
                            tunnel: w340 -> [w377]
                            tunnel: w339 -> [w376]
                            tunnel: [w369] -> w338
                            tunnel: [w362] -> w337
                            stop <- w363 stop-if-true
                            n175 = Concatenate Strings("a1?ia" ("write buffer"), "\r" ("write buffer")) -> (w373:string)
                            n176 = VISA Write(VISA resource name=w377, write buffer=w373, error in (no error)=w376) -> (VISA resource name out=w372:refnum<visa-resource-name>, error out=w371:errorcluster)  [unwired: 1 out]
                            n177 = VISA Read(VISA resource name=w372, byte count=u32 2, error in (no error)=w371) -> (VISA resource name out=w369:refnum<visa-resource-name>, read buffer=w368:string, error out=w362:errorcluster)  [unwired: 1 out]
                            n178 = String To Byte Array(string=w368) -> (unsigned byte array=w367:u8[])
                            n179 = Index Array(array=w367, index=0) -> (element=w365:u8)
                            n180 = Less?(x=w365, y=u8 128) -> (x < y?=w363:bool)
                          }
                          n181 = local read "Init File"() -> (w336:path)
                          n182 = call <vilib>:"Open Config Data.vi"("configuration file path"=w336) -> ("refnum"=w335:T12)  [unwired: 8 in, 2 out]
                          n183 = call-poly <vilib>:"Read Key.vi"("section"="Stage", "key"="Origin", "refnum"=w335) -> ("error out"=w318:errorcluster, "value"=w330:string, "found?"=w317:bool, "refnum out"=w316:T12)  [unwired: 5 in]
                          n184 = Concatenate Strings("a1#p" ("string"), w330, "ug" ("string"), "\r" ("write buffer")) -> (w328:string)
                          n185 = VISA Write(VISA resource name=w338, write buffer=w328, error in (no error)=w337) -> (VISA resource name out=w322:refnum<visa-resource-name>, error out=w321:errorcluster)  [unwired: 1 out]
                          n186 = while {
                            tunnel: w322 -> [w361]
                            tunnel: w321 -> [w360]
                            tunnel: [w353] -> w320
                            tunnel: [w346] -> w319
                            stop <- w347 stop-if-true
                            n187 = Concatenate Strings("a1?ia" ("write buffer"), "\r" ("write buffer")) -> (w357:string)
                            n188 = VISA Write(VISA resource name=w361, write buffer=w357, error in (no error)=w360) -> (VISA resource name out=w356:refnum<visa-resource-name>, error out=w355:errorcluster)  [unwired: 1 out]
                            n189 = VISA Read(VISA resource name=w356, byte count=u32 2, error in (no error)=w355) -> (VISA resource name out=w353:refnum<visa-resource-name>, read buffer=w352:string, error out=w346:errorcluster)  [unwired: 1 out]
                            n190 = String To Byte Array(string=w352) -> (unsigned byte array=w351:u8[])
                            n191 = Index Array(array=w351, index=0) -> (element=w349:u8)
                            n192 = Less?(x=w349, y=u8 128) -> (x < y?=w347:bool)
                          }
                          n193 = call <vilib>:"Close Config Data.vi"("error in (no error)"=w318, "write file if changed (T)"=w317, "refnum"=w316) -> ()  [unwired: 7 in, 2 out]
                          n194 = Concatenate Strings("a1#s0", "\r" ("write buffer")) -> (w323:string)
                          n195 = VISA Write(VISA resource name=w320, write buffer=w323, error in (no error)=w319) -> (VISA resource name out=w327:refnum<visa-resource-name>, error out=w326:errorcluster)  [unwired: 1 out]
                          n196 = VISA Close(VISA resource name=w327, error in (no error)=w326) -> ()  [unwired: 1 out]
                        }
                        frame #2 {
                          n197 = local write "Stage Position"("0" ("Stage Position")) -> ()
                          n198 = local write "Moving"(FALSE ("Moving")) -> ()
                        }
                      }
                    }
                    event "Set Origin": Value Change {
                      w406 = "Origin" ("key")
                      w407 = "Stage" ("section")
                      n199 = event-data() -> ()  [unwired: 1 in, 6 out]
                      n200 = in-place {
                        in-place-border: [w429] -> w417
                        in-place-border: [w434] -> w416
                        w430 = u16 2 items=["None", "Last Bit", "TermChar"] ("Serial Settings:End Mode for Reads")
                        w436 = u16 0 items=["None", "XON/XOFF", "RTS/CTS", "XON/XOFF & RTS/CTS", "DTR/DSR", "XON/XOFF & DTR/DSR"]  # flow control (0:none)
                        w437 = u16 10 items=["1.0"=10, "1.5"=15, "2.0"=20]  # stop bits (10: 1 bit)
                        w438 = FALSE  # Enable Termination Char (T)
                        w439 = u32 2000  # timeout (10sec)
                        w440 = enum16{"None", "Odd", "Even", "Mark", "Space"}."None"  # parity (0:none)
                        w441 = u16 8  # data bits (8)
                        n201 = Type Cast(type=u8 0, x="\r") -> (*(type *) &x=w432:u8)
                        n202 = call-poly "VISA Configure Serial Port"("VISA resource name"=refnum<visa-resource-name> "COM4", "timeout (10sec)"=w439, "Enable Termination\nChar (T)"=w438, "baud rate (9600)"=u32 9600, "data bits (8)"=w441, "parity (0:none)"=w440, "stop bits (10: 1 bit)"=w437, "flow control (0:none)"=w436) -> ("VISA resource name out"=w429:refnum<visa-resource-name>, "error out"=w434:errorcluster)  [unwired: 6 in]
                        n203 = property class="Instr"(reference=w429, "ASRL End In"=w430, "TermChar"=w432) -> ()  [unwired: 1 in, 2 out]
                      }
                      n204 = in-place {
                        in-place-border: w417 -> [w423]
                        in-place-border: w416 -> [w422]
                        in-place-border: [w421] -> w394
                        in-place-border: [w420] -> w395
                        in-place-border: [w418] -> w412
                        n205 = Concatenate Strings("a1?s" ("write buffer"), "\r" ("write buffer")) -> (w426:string)
                        n206 = VISA Write(VISA resource name=w423, write buffer=w426, error in (no error)=w422) -> (VISA resource name out=w427:refnum<visa-resource-name>, error out=w419:errorcluster)  [unwired: 1 out]
                        n207 = VISA Read(VISA resource name=w427, byte count=u32 6, error in (no error)=w419) -> (VISA resource name out=w420:refnum<visa-resource-name>, read buffer=w418:string, error out=w421:errorcluster)  [unwired: 1 out]
                      }
                      n208 = local read "Init File"() -> (w415:path)
                      n209 = call <vilib>:"Open Config Data.vi"("configuration file path"=w415) -> ("refnum"=w414:T12)  [unwired: 8 in, 2 out]
                      n210 = call-poly <vilib>:"Read Key.vi"("section"=w407, "key"=w406, "refnum"=w414) -> ("error out"=w405:errorcluster, "value"=w411:string, "refnum out"=w413:T12)  [unwired: 5 in, 1 out]
                      n211 = Decimal String To Number(string=w411) -> (number=w409:i32)  [unwired: 2 in, 1 out]
                      n212 = Decimal String To Number(string=w412) -> (number=w410:i32)  [unwired: 2 in, 1 out]
                      n213 = Add(x=w410, y=w409) -> (x+y=w403:i32)
                      n214 = Number To Decimal String(number=w403) -> (decimal integer string=w402:string)  [unwired: 1 in]
                      n215 = call-poly <vilib>:"Write Key.vi"("section"=w407, "error in (no error)"=w405, "value"=w402, "key"=w406, "refnum"=w413) -> ("error out"=w404:errorcluster, "refnum out"=w408:T12)  [unwired: 4 in, 1 out]
                      n216 = call <vilib>:"Close Config Data.vi"("error in (no error)"=w404, "refnum"=w408) -> ()  [unwired: 8 in, 2 out]
                      n217 = Concatenate Strings("a1#s0", "\r" ("write buffer")) -> (w397:string)
                      n218 = local write "Stage Position"("0" ("Stage Position")) -> ()
                      n219 = VISA Write(VISA resource name=w395, write buffer=w397, error in (no error)=w394) -> (VISA resource name out=w401:refnum<visa-resource-name>, error out=w400:errorcluster)  [unwired: 1 out]
                      n220 = VISA Close(VISA resource name=w401, error in (no error)=w400) -> ()  [unwired: 1 out]
                    }
                    event "go left Button": Value Change {
                      n221 = event-data() -> ()  [unwired: 1 in, 6 out]
                      n222 = flat-sequence {
                        tunnel: w443 -> [w446]
                        frame #0 {
                          n223 = local write "Moving"(TRUE ("Moving")) -> ()
                        }
                        frame #1 {
                          w452 = u16 2 items=["None", "Last Bit", "TermChar"] ("Serial Settings:End Mode for Reads")
                          w475 = u16 0 items=["None", "XON/XOFF", "RTS/CTS", "XON/XOFF & RTS/CTS", "DTR/DSR", "XON/XOFF & DTR/DSR"]  # flow control (0:none)
                          w474 = u16 10 items=["1.0"=10, "1.5"=15, "2.0"=20]  # stop bits (10: 1 bit)
                          w473 = FALSE  # Enable Termination Char (T)
                          w472 = u32 2000  # timeout (10sec)
                          w471 = enum16{"None", "Odd", "Even", "Mark", "Space"}."None"  # parity (0:none)
                          w470 = u16 8  # data bits (8)
                          n224 = local read "Step length (um)"() -> (w445:dbl)
                          n225 = Type Cast(type=u8 0, x="\r") -> (*(type *) &x=w454:u8)
                          n226 = call-poly "VISA Configure Serial Port"("VISA resource name"=refnum<visa-resource-name> "COM4", "timeout (10sec)"=w472, "Enable Termination\nChar (T)"=w473, "baud rate (9600)"=u32 9600, "data bits (8)"=w470, "parity (0:none)"=w471, "stop bits (10: 1 bit)"=w474, "flow control (0:none)"=w475) -> ("VISA resource name out"=w451:refnum<visa-resource-name>, "error out"=w482:errorcluster)  [unwired: 6 in]
                          n227 = property class="Instr"(reference=w451, "ASRL End In"=w452, "TermChar"=w454) -> ()  [unwired: 1 in, 2 out]
                          n228 = Quotient & Remainder(x=w445, y=w446) -> (x-y*floor(x/y)=w449:dbl)  [unwired: 1 out]
                          n229 = Equal?(x=w449, y=0.0) -> (x = y?=w447:bool)
                          n230 = case shown="False" w447 {
                            frame False {
                              n231 = call "Step too small!"() -> ()  [unwired: 18 in, 2 out]
                            }
                            frame True {
                            }
                          }
                          n232 = Concatenate Strings("a1?s" ("write buffer"), "\r" ("write buffer")) -> (w466:string)
                          n233 = Multiply(x=w445, y=w446) -> (x*y=w450:dbl)
                          n234 = Number To Decimal String(number=w450) -> (decimal integer string=w478:string)  [unwired: 1 in]
                          n235 = Concatenate Strings("a1#p" ("string"), w478, "ug" ("string"), "\r" ("write buffer")) -> (w477:string)
                          n236 = VISA Write(VISA resource name=w451, write buffer=w477, error in (no error)=w482) -> (VISA resource name out=w458:refnum<visa-resource-name>, error out=w457:errorcluster)  [unwired: 1 out]
                          n237 = while {
                            tunnel: w458 -> [w498]
                            tunnel: w457 -> [w497]
                            tunnel: [w490] -> w463
                            tunnel: [w489] -> w462
                            stop <- w483 stop-if-true
                            n238 = Concatenate Strings("a1?ia" ("write buffer"), "\r" ("write buffer")) -> (w494:string)
                            n239 = VISA Write(VISA resource name=w498, write buffer=w494, error in (no error)=w497) -> (VISA resource name out=w493:refnum<visa-resource-name>, error out=w492:errorcluster)  [unwired: 1 out]
                            n240 = VISA Read(VISA resource name=w493, byte count=u32 2, error in (no error)=w492) -> (VISA resource name out=w490:refnum<visa-resource-name>, read buffer=w488:string, error out=w489:errorcluster)  [unwired: 1 out]
                            n241 = String To Byte Array(string=w488) -> (unsigned byte array=w487:u8[])
                            n242 = Index Array(array=w487, index=0) -> (element=w485:u8)
                            n243 = Less?(x=w485, y=u8 128) -> (x < y?=w483:bool)
                          }
                          n244 = VISA Write(VISA resource name=w463, write buffer=w466, error in (no error)=w462) -> (VISA resource name out=w467:refnum<visa-resource-name>, error out=w456:errorcluster)  [unwired: 1 out]
                          n245 = VISA Read(VISA resource name=w467, byte count=u32 6, error in (no error)=w456) -> (VISA resource name out=w460:refnum<visa-resource-name>, read buffer=w459:string, error out=w461:errorcluster)  [unwired: 1 out]
                          n246 = local write "Stage Position"(w459) -> ()
                          n247 = VISA Close(VISA resource name=w460, error in (no error)=w461) -> ()  [unwired: 1 out]
                        }
                        frame #2 {
                          n248 = local write "Moving"(FALSE ("Moving")) -> ()
                        }
                      }
                    }
                    event "Scan Step (um)": Value Change {
                      n249 = event-data() -> ()  [unwired: 1 in, 6 out]
                      n250 = local read "Scan Step (um)"() -> (w500:dbl)
                      n251 = Quotient & Remainder(x=w500, y=w501) -> (x-y*floor(x/y)=w504:dbl)  [unwired: 1 out]
                      n252 = Equal?(x=w504, y=0.0) -> (x = y?=w502:bool)
                      n253 = case shown="False" w502 {
                        frame False {
                          n254 = call "Step too small!"() -> ()  [unwired: 18 in, 2 out]
                        }
                        frame True {
                        }
                      }
                    }
                    event Timeout {
                      n255 = event-data() -> ()  [unwired: 1 in, 3 out]
                    }
                    event Value Change {
                      n256 = event-data() -> ()  [unwired: 1 in, 6 out]
                      n257 = property on="Shutter Control" class="Enum (strict)"() -> ("Value"=w505:T2)  [unwired: 2 in, 2 out]
                      n258 = call <userlib>:"SetShutters.vi"("type"=Shutter_type_typedef."TTL Low", "mode"=w505) -> ()  [unwired: 16 in, 2 out]
                    }
                    event "Exposure Time (s)": Value Change {
                      n259 = event-data() -> ()  [unwired: 1 in, 6 out]
                      n260 = local read "Exposure Time (s)"() -> (w507:sgl)
                      n261 = call <userlib>:"SetExposureTime.vi"("time"=w507) -> ()  [unwired: 1 in, 2 out]
                    }
                    event "Set Temp.": Value Change {
                      n262 = event-data() -> ()  [unwired: 1 in, 6 out]
                      n263 = local read "Set Temp."() -> (w508:dbl)
                      n264 = call <userlib>:"SetTemperature.vi"("temperature"=w508) -> ()  [unwired: 1 in, 2 out]
                    }
                  }
                }
                frame #1 {
                  n265 = local read "OM"() -> (w509:bool)
                  n266 = call <userlib>:"GetStatus.vi"() -> ("status"=w514:T1)  [unwired: 3 in, 2 out]
                  n267 = local read "Live View"() -> (w510:bool)
                  n268 = Equal?(x=w514, y=Error_Code_Enum_typedef."DRV_IDLE" ("status")) -> (x = y?=w512:bool)
                  n269 = case shown="True" w509 {
                    frame False {
                      w515 = TRUE ("Visible")
                      w516 = FALSE ("Visible")
                      n270 = property on="new picture" class="Pict"("Visible"=w516) -> ()  [unwired: 2 in, 2 out]
                      n271 = property on="sharp" class="DigNum (strict)"("Visible"=w516) -> ()  [unwired: 2 in, 2 out]
                      n272 = property on="bright" class="DigNum (strict)"("Visible"=w516) -> ()  [unwired: 2 in, 2 out]
                      n273 = property on="gamma" class="DigNum (strict)"("Visible"=w516) -> ()  [unwired: 2 in, 2 out]
                      n274 = property on="contrast" class="DigNum (strict)"("Visible"=w516) -> ()  [unwired: 2 in, 2 out]
                      n275 = property on="Red Gain" class="Slide (strict)"("Visible"=w516) -> ()  [unwired: 2 in, 2 out]
                      n276 = property on="Blue Gain" class="Slide (strict)"("Visible"=w516) -> ()  [unwired: 2 in, 2 out]
                      n277 = property on="Green Gain" class="Slide (strict)"("Visible"=w516) -> ()  [unwired: 2 in, 2 out]
                      n278 = property on="Gain?" class="Bool (strict)"("Visible"=w516) -> ()  [unwired: 2 in, 2 out]
                      n279 = property on="ET Labelµ" class="DigNum (strict)"("Visible"=w516) -> ()  [unwired: 2 in, 2 out]
                      n280 = property on="Wavelength" class="Slide (strict)"("Visible"=w515) -> ()  [unwired: 2 in, 2 out]
                      n281 = property on="Exposure Time:" class="Slide (strict)"("Visible"=w516) -> ()  [unwired: 2 in, 2 out]
                      n282 = property on="Bandwidth" class="DigNum (strict)"("Visible"=w515) -> ()  [unwired: 2 in, 2 out]
                    }
                    frame True {
                      w517 = FALSE ("Visible")
                      w522 = TRUE ("Visible")
                      w526 = 4 ("y")
                      w555 = 1
                      # "We skip the first 256 bytes,\nand show the first Row only."
                      n283 = property on="contrast" class="DigNum (strict)"("Visible"=w522) -> ()  [unwired: 2 in, 2 out]
                      n284 = property on="bright" class="DigNum (strict)"("Visible"=w522) -> ()  [unwired: 2 in, 2 out]
                      n285 = property on="sharp" class="DigNum (strict)"("Visible"=w522) -> ()  [unwired: 2 in, 2 out]
                      n286 = property on="new picture" class="Pict"("Visible"=w522) -> ()  [unwired: 2 in, 2 out]
                      n287 = Divide(x=1920, y=w526) -> (x/y=w518:dbl)
                      n288 = Divide(x=2560, y=w526) -> (x/y=w519:dbl)
                      n289 = Compound Arithmetic op=MULTIPLY(w519, w518, 3.0 ("y")) -> (w520:dbl)
                      n290 = property on="gamma" class="DigNum (strict)"("Visible"=w522) -> ()  [unwired: 2 in, 2 out]
                      n291 = property on="Red Gain" class="Slide (strict)"("Visible"=w522) -> ()  [unwired: 2 in, 2 out]
                      n292 = property on="Gain?" class="Bool (strict)"("Visible"=w522) -> ()  [unwired: 2 in, 2 out]
                      n293 = Add(x=w520, y=256.0) -> (x+y=w523:dbl)
                      n294 = Initialize Array(u8 0, w523) -> (w524:u8[])
                      n295 = property on="Green Gain" class="Slide (strict)"("Visible"=w522) -> ()  [unwired: 2 in, 2 out]
                      n296 = Multiply(x="Exposure Time:", y=1) -> (x*y=→"ET Labelµ":dbl)
                      n297 = property on="Blue Gain" class="Slide (strict)"("Visible"=w522) -> ()  [unwired: 2 in, 2 out]
                      n298 = Multiply(x=w523, y=1) -> (x*y=w556:dbl)
                      n299 = Multiply(x="Exposure Time:", y=20) -> (x*y=w560:dbl)
                      n300 = dll-call lib="D:/All users/PoSheng/src/lib/SSClassic_USBCamera_SDK.dll" fn="SSClassicUSB_SetExposureTime" ("CCD_USBCamera_SDK.dll:CCDUSB_SetExposureTime")("Arg1"=1, "Arg2"=w560) -> (error out=w543:errorcluster)  [unwired: 6 in, 1 out]
                      n301 = property on="Exposure Time:" class="Slide (strict)"("Visible"=w522) -> ()  [unwired: 2 in, 2 out]
                      n302 = property on="ET Labelµ" class="DigNum (strict)"("Visible"=w522) -> ()  [unwired: 2 in, 2 out]
                      n303 = case shown="True" "Gain?" {
                        tunnel: w543 -> [w565 w571]
                        tunnel: [w565 w570] -> w536
                        tunnel: 1 ("deviceID") -> [_ w569]
                        tunnel: "Red Gain" -> [_ w568]
                        tunnel: "Green Gain" -> [_ w567]
                        tunnel: "Blue Gain" -> [_ w566]
                        frame False {
                        }
                        frame True {
                          n304 = dll-call lib="D:/All users/PoSheng/src/lib/SSClassic_USBCamera_SDK.dll" fn="SSClassicUSB_SetGains" ("CCD_USBCamera_SDK.dll:CCDUSB_SetExposureTime")(error in=w571, "deviceID"=w569, "redGain"=w568, "greenGain"=w567, "blueGain"=w566) -> (error out=w570:errorcluster)  [unwired: 7 in, 1 out]
                        }
                      }
                      n305 = property on="Wavelength" class="Slide (strict)"("Visible"=w517) -> ()  [unwired: 2 in, 2 out]
                      n306 = property on="Bandwidth" class="DigNum (strict)"("Visible"=w517) -> ()  [unwired: 2 in, 2 out]
                      n307 = dll-call lib="D:/All users/PoSheng/src/lib/SSClassic_USBCamera_SDK.dll" fn="SSClassicUSB_SetGamma" ("CCD_USBCamera_SDK.dll:CCDUSB_GetCurrentFrame")(error in=w536, "deviceID"=1, "gamma"="gamma", "contrast"="contrast", "bright"="bright", "sharp"="sharp") -> (error out=w535:errorcluster)  [unwired: 8 in, 1 out]
                      n308 = dll-call lib="D:/All users/PoSheng/src/lib/SSClassic_USBCamera_SDK.dll" fn="SSClassicUSB_GetCurrentFrame" ("CCD_USBCamera_SDK.dll:CCDUSB_GetCurrentFrame")(error in=w535, "Arg1"=w555, "Arg2"=w555, "Arg3"=w524) -> (error out=w544:errorcluster, "ReturnValue"=w564:i64)  [unwired: 5 in, 1 out]
                      n309 = dll-call lib="LabVIEW" fn="MoveBlock"(error in=w544, "src"=w564, "dst"=w524, "size"=w556) -> ("dst"=w549:u8[])  [unwired: 5 in, 2 out]
                      n310 = Split 1D Array(array=w549, index=256 ("y")) -> (second subarray=w554:u8[])  [unwired: 1 out]
                      n311 = Decimate 1D Array(w554) -> (w551:u8[], w552:u8[], w545:u8[])
                      n312 = Join Numbers(hi=w552, lo=w551) -> ((hi.lo)=w553:u16[])
                      n313 = Join Numbers(hi=w545, lo=w553) -> ((hi.lo)=w550:u32[])
                      n314 = Reshape Array(w550, w518, w519) -> (w548:u32[][])
                      n315 = call "array_to_pixmap.vi"("photoarray"=w548) -> ("pixmap out"=w547:T13)  [unwired: 9 in, 1 out]
                      n316 = call <vilib>:"Draw Flattened Pixmap.vi"("image data"=w547) -> ("new picture"=→"new picture":picture)  [unwired: 8 in]
                    }
                  }
                  n317 = And(x=w512, y=w510) -> (x .and. y?=w511:bool)
                  n318 = case shown="True" w511 {
                    frame False {
                    }
                    frame True {
                      n319 = flat-sequence {
                        tunnel: [w574] -> w573
                        tunnel: w573 -> [w575]
                        tunnel: [w575] -> w572
                        tunnel: w572 -> [w581]
                        frame #0 {
                          n320 = call <userlib>:"StartAcquisition.vi"() -> ("DLL error code"=w574:u32)  [unwired: 2 in, 1 out]
                        }
                        frame #1 {
                          n321 = while {
                            stop <- w578 stop-if-true
                            n322 = call <userlib>:"GetStatus.vi"() -> ("status"=w576:T1)  [unwired: 3 in, 2 out]
                            n323 = Equal?(x=w576, y=Error_Code_Enum_typedef."DRV_IDLE" ("status")) -> (x = y?=w578:bool)
                          }
                        }
                        frame #2 {
                          n324 = Equal?(x=w581, y=u32 20002) -> (x = y?=w579:bool)
                          n325 = case shown="True" w579 {
                            frame False {
                            }
                            frame True {
                              w583 = 512
                              n326 = To Long Integer(number=w583) -> (32bit integer=w585:i32)
                              n327 = To Long Integer(number=w583) -> (32bit integer=w584:i32)
                              n328 = Multiply(x=w585, y=w584) -> (x*y=w589:i32)
                              n329 = call <userlib>:"GetAcquiredData.vi"("size"=w589) -> ("array"=w587:i32[])  [unwired: 2 in, 2 out]
                              n330 = Multiply(x=1, y=w587) -> (x*y=w586:i32[])
                              n331 = Reshape Array(w586, w584, w585) -> (→"Left Graph":i32[][])
                            }
                          }
                        }
                      }
                    }
                  }
                }
                frame #2 {
                  n332 = call <userlib>:"GetTemperature.vi"() -> ("status"=w592:T1, "temperature"=w593:i32)  [unwired: 4 in, 2 out]
                  n333 = Equal?(x=w592, y=Error_Code_Enum_typedef."DRV_TEMPERATURE_STABILIZED") -> (x = y?=w590:bool)
                  n334 = case shown="True" w590 {
                    frame False {
                      n335 = local write "Cooler"(FALSE ("Cooler")) -> ()
                    }
                    frame True {
                      n336 = local write "Cooler"(TRUE ("Cooler")) -> ()
                    }
                  }
                  n337 = local write "temp. status 2"(w592) -> ()
                  n338 = local write "Temp"(w593) -> ()
                }
                frame #3 {
                  n339 = call <userlib>:"GetStatus.vi"() -> ("status"=w596:T1)  [unwired: 3 in, 2 out]
                  n340 = local write "Status"(w596) -> ()
                }
              }
              n341 = local read "Shut Down"() -> (w214:bool)
              n342 = Or(x="Scan Start", y=w214) -> (x .or. y?=w213:bool)
              "Numeric 2" <- w218
            }
          }
          frame #1 {
            w610 = TRUE ("Visible")
            w609 = T11."Disabled and Grayed Out" ("Disabled")
            n343 = property on="Right Graph" class="IntGraph (strict)"("Caption.Text"="Object Image") -> ()  [unwired: 2 in, 2 out]
            n344 = property on="Go back after scan" class="Bool (strict)"("DisabledEnum"=w609) -> ()  [unwired: 2 in, 2 out]
            n345 = property on="Shutter Control" class="Enum (strict)"("DisabledEnum"=w609) -> ()  [unwired: 2 in, 2 out]
            n346 = property on="go left Button" class="Bool"("DisabledEnum"=w609) -> ()  [unwired: 2 in, 2 out]
            n347 = property on="HSS (MHz)" class="Ring (strict)"("DisabledEnum"=w609) -> ()  [unwired: 2 in, 2 out]
            n348 = property on="VSS (s)" class="Ring (strict)"("DisabledEnum"=w609) -> ()  [unwired: 2 in, 2 out]
            n349 = property on="Live View" class="Bool (strict)"("DisabledEnum"=w609) -> ()  [unwired: 2 in, 2 out]
            n350 = property on="Current \nScan Frame" class="DigNum (strict)"("Visible"=w610) -> ()  [unwired: 2 in, 2 out]
            n351 = property on="Scan Abort" class="Bool"("DisabledEnum"=T11."Enabled" ("Disabled")) -> ()  [unwired: 2 in, 2 out]
            n352 = property on="Total \nScan Frame" class="DigNum (strict)"("Visible"=w610) -> ()  [unwired: 2 in, 2 out]
            n353 = property on="Exposure Time (s)" class="DigNum (strict)"("DisabledEnum"=w609) -> ()  [unwired: 2 in, 2 out]
            n354 = property on="Step length (um)" class="DigNum (strict)"("DisabledEnum"=w609) -> ()  [unwired: 2 in, 2 out]
            n355 = property on="Take shot" class="Bool (strict)"("DisabledEnum"=w609) -> ()  [unwired: 2 in, 2 out]
            n356 = property on="Scan Length (mm)" class="DigNum (strict)"("DisabledEnum"=w609) -> ()  [unwired: 2 in, 2 out]
            n357 = property on="Scan Start" class="Bool"("DisabledEnum"=w609) -> ()  [unwired: 2 in, 2 out]
            n358 = property on="go right Button" class="Bool"("DisabledEnum"=w609) -> ()  [unwired: 2 in, 2 out]
            n359 = property on="Scan Step (um)" class="DigNum (strict)"("DisabledEnum"=w609) -> ()  [unwired: 2 in, 2 out]
            n360 = invoke on="Right Graph" class="IntGraph (strict)" method="Reinit To Default"() -> ()  [unwired: 3 in, 3 out]
            n361 = local write "Right Graph"(i32[][] [] ("Right Graph")) -> ()
            n362 = dll-call lib="D:/All users/PoSheng/src/lib/SSClassic_USBCamera_SDK.dll" fn="SSClassicUSB_StopCameraEngine" ("CCD_USBCamera_SDK.dll:CCDUSB_StopCameraEngine")() -> (error out=w597:errorcluster)  [unwired: 4 in, 1 out]
            n363 = dll-call lib="D:/All users/PoSheng/src/lib/SSClassic_USBCamera_SDK.dll" fn="SSClassicUSB_UnInitDevice" ("CCD_USBCamera_SDK.dll:CCDUSB_UnInitDevice")(error in=w597) -> ()  [unwired: 3 in, 2 out]
            n364 = in-place {
              in-place-border: [w625] -> w607
              in-place-border: [w630] -> w606
              w626 = u16 2 items=["None", "Last Bit", "TermChar"] ("Serial Settings:End Mode for Reads")
              w632 = u16 0 items=["None", "XON/XOFF", "RTS/CTS", "XON/XOFF & RTS/CTS", "DTR/DSR", "XON/XOFF & DTR/DSR"]  # flow control (0:none)
              w633 = u16 10 items=["1.0"=10, "1.5"=15, "2.0"=20]  # stop bits (10: 1 bit)
              w634 = FALSE  # Enable Termination Char (T)
              w635 = u32 2000  # timeout (10sec)
              w636 = enum16{"None", "Odd", "Even", "Mark", "Space"}."None"  # parity (0:none)
              w637 = u16 8  # data bits (8)
              n365 = Type Cast(type=u8 0, x="\r") -> (*(type *) &x=w628:u8)
              n366 = call-poly "VISA Configure Serial Port"("VISA resource name"=refnum<visa-resource-name> "COM4", "timeout (10sec)"=w635, "Enable Termination\nChar (T)"=w634, "baud rate (9600)"=u32 9600, "data bits (8)"=w637, "parity (0:none)"=w636, "stop bits (10: 1 bit)"=w633, "flow control (0:none)"=w632) -> ("VISA resource name out"=w625:refnum<visa-resource-name>, "error out"=w630:errorcluster)  [unwired: 6 in]
              n367 = property class="Instr"(reference=w625, "ASRL End In"=w626, "TermChar"=w628) -> ()  [unwired: 1 in, 2 out]
            }
            n368 = in-place {
              in-place-border: w607 -> [w619]
              in-place-border: w606 -> [w618]
              in-place-border: [w617] -> w604
              in-place-border: [w616] -> w605
              in-place-border: [w614] -> w603
              n369 = Concatenate Strings("a1?s" ("write buffer"), "\r" ("write buffer")) -> (w622:string)
              n370 = VISA Write(VISA resource name=w619, write buffer=w622, error in (no error)=w618) -> (VISA resource name out=w623:refnum<visa-resource-name>, error out=w615:errorcluster)  [unwired: 1 out]
              n371 = VISA Read(VISA resource name=w623, byte count=u32 6, error in (no error)=w615) -> (VISA resource name out=w616:refnum<visa-resource-name>, read buffer=w614:string, error out=w617:errorcluster)  [unwired: 1 out]
            }
            n372 = VISA Close(VISA resource name=w605, error in (no error)=w604) -> ()  [unwired: 1 out]
            n373 = String Length(string=w603) -> (length=w601:i32)
            n374 = Subtract(x=w601, y=1) -> (x-y=w599:i32)
            n375 = String Subset(string=w603, offset (0)=0, length (rest)=w599) -> (substring=w598:string)
            n376 = local read "Shut Down"() -> (w613:bool)
            n377 = case shown="True" w613 {
              frame False {
              }
              frame True {
                n378 = local write "Scan Length (mm)"(0.0 ("Scan Length (mm)")) -> ()
              }
            }
          }
          frame #2 {
            n379 = in-place {
              in-place-border: [w681] -> _
              in-place-border: [w664] -> w642
              in-place-border: [w655] -> w643
              in-place-border: w641 -> [w654]
              in-place-border: w640 -> [w650]
              w659 = 1000.0  # mm to um
              w697 = u16 0 items=["None", "XON/XOFF", "RTS/CTS", "XON/XOFF & RTS/CTS", "DTR/DSR", "XON/XOFF & DTR/DSR"]  # flow control (0:none)
              w698 = u16 10 items=["1.0"=10, "1.5"=15, "2.0"=20]  # stop bits (10: 1 bit)
              w699 = FALSE  # Enable Termination Char (T)
              w700 = u32 2000  # timeout (10sec)
              w701 = enum16{"None", "Odd", "Even", "Mark", "Space"}."None"  # parity (0:none)
              w702 = u16 8  # data bits (8)
              n380 = local read "Scan Length (mm)"() -> (w647:dbl)
              n381 = property on="Right Graph" class="IntGraph (strict)"("ActXScl"=0 ("Active X Scale"), "XScale.ScaleFit"=u8 0 ("X Scale.Scale Fit"), "XScale.Maximum"=w647, "XScale.Minimum"=0.0 ("X Scale.Range:Minimum")) -> ()  [unwired: 2 in, 2 out]
              n382 = Initialize Array(sgl 400.0 ("element")) -> (w676:sgl[])  [unwired: 1 in]
              n383 = call-poly "VISA Configure Serial Port"("VISA resource name"=refnum<visa-resource-name> "COM4", "timeout (10sec)"=w700, "Enable Termination\nChar (T)"=w699, "baud rate (9600)"=u32 9600, "data bits (8)"=w702, "parity (0:none)"=w701, "stop bits (10: 1 bit)"=w698, "flow control (0:none)"=w697) -> ("VISA resource name out"=w695:refnum<visa-resource-name>, "error out"=w694:errorcluster)  [unwired: 6 in]
              n384 = for {
                N: 512 -> [_]
                shift-right: [w797] -> w677
                shift-left: w676 -> [w798]
                i -> [w796]
                n385 = Multiply(x=w796, y=sgl -1.5446) -> (x*y=w794:sgl)
                n386 = Add(x=sgl 1105.4, y=w794) -> (x+y=w792:sgl)
                n387 = Insert Into Array(array=w798, index=w796, new element=w792) -> (w797:sgl[])
              }
              n388 = local read "Exposure Time (s)"() -> (w671:sgl)
              n389 = Reverse 1D Array(array=w677) -> (reversed array=w655:sgl[])
              n390 = local read "Scan Step (um)"() -> (w658:dbl)
              n391 = Compound Arithmetic op=MULTIPLY(w671, sgl 1000.0 ("y"), sgl 1.5 ("value")) -> (w668:sgl)
              n392 = Array Max & Min(array=w655) -> (max value=w678:sgl, min value=w672:sgl)  [unwired: 2 out]
              n393 = Subtract(x=w678, y=w672) -> (x-y=w679:sgl)
              n394 = control-ref of="Waveform Graph"() -> (w667:refnum<vi>)
              n395 = Divide(x=w658, y=w659) -> (x/y=w646:dbl)
              n396 = Quotient & Remainder(x=w647, y=w646) -> (floor(x/y)=w649:dbl)  [unwired: 1 out]
              n397 = local write "Total \nScan Frame"(w649) -> ()
              n398 = Multiply(x=w650, y=w658) -> (x*y=w651:dbl)
              n399 = for {
                N: w649 -> [_]
                tunnel: w695 -> [w737]
                tunnel: w694 -> [w736]
                tunnel: [w734] -> w693
                tunnel: [w733] -> w692
                tunnel: [w727] -> w686 mode=indexing
                tunnel: w651 -> [w735]
                tunnel: w668 -> [w732]
                tunnel: [w730] -> w666
                shift-right: [w723] -> _
                shift-left: i32[][] [] -> [w724]
                i -> [w731]
                stop <- w730 stop-if-true
                n400 = stacked-sequence {
                  tunnel: w737 -> [_ w754 _]
                  tunnel: w736 -> [_ w753 _]
                  tunnel: [_ w747 _] -> w734
                  tunnel: [_ _ w760] -> w727
                  tunnel: w735 -> [_ w748 w758]
                  tunnel: [_ w746 _] -> w733
                  tunnel: w732 -> [_ _ w759]
                  tunnel: [w742 _ _] -> w730
                  frame #0 {
                    n401 = event shown="[1] \"Scan Abort\": Value Change" {
                      selector: _ -> [_ _]
                      dyn-events: _ -> [_ _]
                      timeout: 0 -> [_ _]
                      tunnel: [FALSE TRUE] -> w742
                      event Timeout {
                        n402 = event-data() -> ()  [unwired: 1 in, 3 out]
                      }
                      event "Scan Abort": Value Change {
                        n403 = event-data() -> ()  [unwired: 1 in, 6 out]
                      }
                    }
                  }
                  frame #1 {
                    n404 = Number To Decimal String(number=w748) -> (decimal integer string=w749:string)  [unwired: 1 in]
                    n405 = Concatenate Strings("a1#p" ("string"), w749, "ug" ("string"), "\r" ("write buffer")) -> (w755:string)
                    n406 = VISA Write(VISA resource name=w754, write buffer=w755, error in (no error)=w753) -> (VISA resource name out=w747:refnum<visa-resource-name>, error out=w746:errorcluster)  [unwired: 1 out]
                  }
                  frame #2 {
                    n407 = flat-sequence {
                      tunnel: [w767] -> w761
                      tunnel: w758 -> [w766]
                      tunnel: w761 -> [w769]
                      tunnel: [w769] -> w757
                      tunnel: w759 -> [w768]
                      tunnel: w757 -> [w777]
                      tunnel: [w777] -> w756
                      tunnel: w756 -> [w781]
                      tunnel: [w778] -> w760
                      frame #0 {
                        n408 = call <userlib>:"StartAcquisition.vi"() -> ("DLL error code"=w767:u32)  [unwired: 2 in, 1 out]
                        n409 = Divide(x=w766, y=200.0) -> (x/y=w763:dbl)
                        n410 = Multiply(x=u32 750 ("milliseconds to wait"), y=w763) -> (x*y=w762:dbl)
                        n411 = Wait (ms)(milliseconds to wait=w762) -> ()  [unwired: 1 out]
                      }
                      frame #1 {
                        n412 = while {
                          tunnel: w768 -> [w770]
                          stop <- w771 stop-if-true
                          n413 = flat-sequence {
                            tunnel: [w772] -> w771
                            tunnel: w770 -> [w775]
                            frame #0 {
                              n414 = call <userlib>:"GetStatus.vi"() -> ("status"=w773:T1)  [unwired: 3 in, 2 out]
                              n415 = Equal?(x=w773, y=Error_Code_Enum_typedef."DRV_IDLE" ("status")) -> (x = y?=w772:bool)
                            }
                            frame #1 {
                              n416 = Wait (ms)(milliseconds to wait=w775) -> ()  [unwired: 1 out]
                            }
                          }
                        }
                      }
                      frame #2 {
                        n417 = call <vilib>:"High Resolution Relative Seconds.vi"() -> ("relative seconds"=→"relative seconds":dbl)
                      }
                      frame #3 {
                        n418 = Equal?(x=w781, y=u32 20002) -> (x = y?=w779:bool)
                        n419 = case shown="True" w779 {
                          tunnel: [i32[][] [] w783] -> w778
                          frame False {
                          }
                          frame True {
                            w784 = 512
                            n420 = To Long Integer(number=w784) -> (32bit integer=w786:i32)
                            n421 = To Long Integer(number=w784) -> (32bit integer=w785:i32)
                            n422 = Multiply(x=w786, y=w785) -> (x*y=w790:i32)
                            n423 = call <userlib>:"GetAcquiredData.vi"("size"=w790) -> ("array"=w788:i32[])  [unwired: 2 in, 2 out]
                            n424 = Multiply(x=1, y=w788) -> (x*y=w787:i32[])
                            n425 = Reshape Array(w787, w785, w786) -> (w783:i32[][])
                            n426 = local write "Left Graph"(w783) -> ()
                          }
                        }
                      }
                      frame #4 {
                        n427 = call <vilib>:"High Resolution Relative Seconds.vi"() -> ("relative seconds"=→"relative seconds 2":dbl)
                      }
                    }
                  }
                }
                n428 = Add(x=w731, y=1) -> (x+y=w729:i32)
                n429 = local write "Current \nScan Frame"(w729) -> ()
                n430 = for {
                  N: 512 -> [_]
                  tunnel: w727 -> [w741]
                  tunnel: [w738] -> w725 mode=indexing
                  i -> [w740]
                  n431 = Index Array(array=w741, index (row)=w740) -> (element=w739:i32[])  [unwired: 1 in]
                  n432 = Add Array Elements(numeric array=w739) -> (sum=w738:i32)
                }
                n433 = Build Array (concatenate)(w724, w725) -> (w723:i32[][])
                n434 = Transpose 2D Array(2D array=w723) -> (transposed array=w722:i32[][])
                n435 = local write "Right Graph"(w722) -> ()
              }
              n436 = Divide(x=w679, y=sgl 512.0) -> (x/y=w673:sgl)
              n437 = property on="Right Graph" class="IntGraph (strict)"("XScale.Offset"=0.0 ("X Scale.Offset and Multiplier:Offset"), "XScale.Multiplier"=w646, "XScale.NameLbl.Text"="X (mm)" ("X Scale.Name Label.Text")) -> ()  [unwired: 2 in, 2 out]
              n438 = property on="Property Node" class="WFGraph (strict)"(reference=w667, "XScale.Multiplier"=w673, "XScale.Offset"=w672) -> ()  [unwired: 1 in, 2 out]
              n439 = property on="Left Graph" class="IntGraph (strict)"("XScale.Multiplier"=w673, "XScale.Offset"=w672) -> ()  [unwired: 2 in, 2 out]
              n440 = Initialize Array(0 ("element")) -> (w683:i32[][][])  [unwired: 3 in]
              n441 = for {
                N: 512 -> [_]
                tunnel: w686 -> [w721]
                shift-right: [w718] -> w664
                shift-left: w683 -> [w717]
                i -> [w715]
                n442 = Index Array(array=w721, index (dim 1)=w715) -> (element=w720:i32[][])  [unwired: 2 in]
                n443 = property on="Constructing data" class="Slide (strict)"("Visible"=TRUE) -> ()  [unwired: 2 in, 2 out]
                n444 = Transpose 2D Array(2D array=w720) -> (transposed array=w719:i32[][])
                n445 = Insert Into Array(array=w717, index (dim 1)=w715, new element=w719) -> (w718:i32[][][])  [unwired: 2 in]
                "Constructing data" <- w715
              }
              n446 = property on="Wavelength" class="Slide (strict)"("Scale.MarkerVals[]"=w655) -> ()  [unwired: 2 in, 2 out]
              n447 = case shown="False" w666 {
                tunnel: [w711 w713] -> w665
                tunnel: w646 -> [_ w712]
                frame False {
                  n448 = local read "Scan Length (mm)"() -> (w711:dbl)
                }
                frame True {
                  n449 = local read "Current \nScan Frame"() -> (w714:dbl)
                  n450 = Multiply(x=w714, y=w712) -> (x*y=w713:dbl)
                }
              }
              n451 = Multiply(x=w665, y=1000) -> (x*y=w687:dbl)
              n452 = Index Array(array=w664, index (dim 0)=175 ("index (page)")) -> (element=w662:i32[][])  [unwired: 2 in]
              n453 = Number To Decimal String(number=w687) -> ()  [unwired: 1 in, 1 out]
              n454 = local write "Right Graph"(w662) -> ()
              n455 = Concatenate Strings("a1#a" ("string"), w654, "g" ("string"), "\r" ("write buffer")) -> (w688:string)
              n456 = case shown="True" "Go back after scan" {
                tunnel: w693 -> [w705 w710]
                tunnel: w692 -> [w704 w709]
                tunnel: [w704 w708] -> w691
                tunnel: [w705 w707] -> w690
                tunnel: w688 -> [_ w706]
                frame False {
                }
                frame True {
                  n457 = VISA Write(VISA resource name=w710, write buffer=w706, error in (no error)=w709) -> (VISA resource name out=w707:refnum<visa-resource-name>, error out=w708:errorcluster)  [unwired: 1 out]
                }
              }
              n458 = VISA Close(VISA resource name=w690, error in (no error)=w691) -> (error out=w681:errorcluster)
            }
          }
          frame #3 {
            n459 = flat-sequence {
              tunnel: w802 -> [w810]
              tunnel: w801 -> [w809]
              tunnel: [w808] -> w799
              tunnel: [w947] -> w800
              tunnel: w799 -> [w947]
              frame #0 {
                w806 = TRUE ("Visible")
                w805 = FALSE ("Visible")
                w803 = T11."Disabled and Grayed Out" ("Disabled")
                w807 = T11."Enabled" ("Disabled")
                n460 = invoke on="X" class="DigNum (strict)" method="Reinit To Default"() -> ()  [unwired: 3 in, 3 out]
                n461 = invoke on="Left Graph" class="IntGraph (strict)" method="Reinit To Default"() -> ()  [unwired: 3 in, 3 out]
                n462 = property on="Constructing data" class="Slide (strict)"("Visible"=w805) -> ()  [unwired: 2 in, 2 out]
                n463 = property on="Total \nScan Frame" class="DigNum (strict)"("Visible"=w805) -> ()  [unwired: 2 in, 2 out]
                n464 = property on="Current \nScan Frame" class="DigNum (strict)"("Visible"=w805) -> ()  [unwired: 2 in, 2 out]
                n465 = property on="Bandwidth" class="DigNum (strict)"("DisabledEnum"=w807) -> ()  [unwired: 2 in, 2 out]
                n466 = property on="path" class="Path"("DisabledEnum"=w807) -> ()  [unwired: 2 in, 2 out]
                n467 = property on="Wavelength" class="Slide (strict)"("DisabledEnum"=w807) -> ()  [unwired: 2 in, 2 out]
                n468 = property on="Waveform Graph" class="WFGraph (strict)"("DisabledEnum"=w807) -> ()  [unwired: 2 in, 2 out]
                n469 = property on="Scan again" class="Bool"("DisabledEnum"=w807) -> ()  [unwired: 2 in, 2 out]
                n470 = property on="Save File" class="Bool (strict)"("DisabledEnum"=w807) -> ()  [unwired: 2 in, 2 out]
                n471 = invoke on="Y" class="DigNum (strict)" method="Reinit To Default"() -> ()  [unwired: 3 in, 3 out]
                n472 = property on="Y" class="DigNum (strict)"("Visible"=w806) -> ()  [unwired: 2 in, 2 out]
                n473 = property on="X" class="DigNum (strict)"("Visible"=w806) -> ()  [unwired: 2 in, 2 out]
                n474 = property on="Right Graph" class="IntGraph (strict)"("XScale.ScaleFit"=u8 2 ("X Scale.Scale Fit")) -> ()  [unwired: 2 in, 2 out]
                n475 = property on="Set Temp." class="DigNum (strict)"("DisabledEnum"=w803) -> ()  [unwired: 2 in, 2 out]
                n476 = property on="Scan Abort" class="Bool"("DisabledEnum"=w803) -> ()  [unwired: 2 in, 2 out]
              }
              frame #1 {
                n477 = in-place {
                  in-place-border: w810 -> [w815]
                  in-place-border: [w814] -> w808
                  in-place-border: [w813] -> _
                  in-place-border: w809 -> [w812]
                  in-place-border: w810 -> [w811]
                  n478 = while {
                    tunnel: w815 -> [w838]
                    tunnel: ["Shut Down"] -> w814
                    tunnel: ["Scan again"] -> w813
                    tunnel: w812 -> [w830]
                    tunnel: w811 -> [w829]
                    stop <- w832 stop-if-true
                    n479 = Subtract(x="Wavelength", y=1105.4) -> (x-y=w820:dbl)
                    n480 = event shown="[0] \"Right Graph\": Mouse Down" {
                      selector: _ -> [_ _]
                      dyn-events: _ -> [_ _]
                      timeout: 10 -> [_ _]
                      tunnel: w838 -> [w909 _]
                      tunnel: [w896 w943] -> w825
                      tunnel: [w895 w942] -> w824
                      event "Right Graph": Mouse Down {
                        # "<-- asymmetry"
                        # "Needed because panel (0,0) is at TOP left rather than bottom left."
                        n481 = event-data() -> ("Coords"=w912:T14)  [unwired: 1 in, 2 out]
                        n482 = control-ref of="Right Graph"() -> (w911:refnum<vi>)
                        n483 = property on="Property Node" class="IntensityGraph (strict)"(reference=w911) -> ("X Scale.Range:Maximum"=w918:dbl, "X Scale.Range:Minimum"=w917:dbl, "Plot Area:Size:Width"=w916:u32, "Plot Area:Position:Left"=w915:i32)  [unwired: 1 in, 2 out]
                        n484 = property on="Property Node" class="IntensityGraph (strict)"(reference=w911) -> ("Y Scale.Range:Maximum"=w941:dbl, "Y Scale.Range:Minimum"=w936:dbl, "Plot Area:Size:Height"=w934:u32, "Plot Area:Position:Top"=w927:i32)  [unwired: 1 in, 2 out]
                        n485 = Unbundle By Name(w912) -> ("Horizontal"=w914:i32)
                        n486 = Unbundle By Name(w912) -> ("Vertical"=w940:i32)
                        n487 = To Double Precision Float(number=w914) -> (double precision float=w922:dbl)
                        n488 = To Double Precision Float(number=w927) -> (double precision float=w932:dbl)
                        n489 = To Double Precision Float(number=w940) -> (double precision float=w933:dbl)
                        n490 = To Double Precision Float(number=w915) -> (double precision float=w923:dbl)
                        n491 = To Double Precision Float(number=w916) -> (double precision float=w926:dbl)
                        n492 = To Double Precision Float(number=w934) -> (double precision float=w928:dbl)
                        n493 = Subtract(x=w922, y=w923) -> (x-y=w913:dbl)
                        n494 = Subtract(x=w933, y=w932) -> (x-y=w935:dbl)
                        n495 = Subtract(x=w928, y=w935) -> (x-y=w931:dbl)
                        n496 = In Range and Coerce(upper limit=w926, x=w913, lower limit=0.0) -> (coerced(x)=w925:dbl)  [unwired: 1 out]
                        n497 = In Range and Coerce(upper limit=w928, x=w931, lower limit=0.0) -> (coerced(x)=w929:dbl)  [unwired: 1 out]
                        n498 = Subtract(x=w918, y=w917) -> (x-y=w919:dbl)
                        n499 = Divide(x=w925, y=w926) -> (x/y=w920:dbl)
                        n500 = Subtract(x=w941, y=w936) -> (x-y=w939:dbl)
                        n501 = Divide(x=w929, y=w928) -> (x/y=w938:dbl)
                        n502 = Multiply(x=w919, y=w920) -> (x*y=w921:dbl)
                        n503 = Multiply(x=w939, y=w938) -> (x*y=w937:dbl)
                        n504 = property on="Right Graph" class="IntGraph (strict)"() -> ("XScale.Multiplier"=w904:dbl, "XScale.Offset"=w906:dbl, "YScale.Multiplier"=w899:dbl, "YScale.Offset"=w901:dbl)  [unwired: 2 in, 2 out]
                        n505 = Add(x=w921, y=w917) -> (x+y=w896:dbl)
                        n506 = Add(x=w937, y=w936) -> (x+y=w895:dbl)
                        n507 = Subtract(x=w895, y=w901) -> (x-y=w900:dbl)
                        n508 = Subtract(x=w896, y=w906) -> (x-y=w905:dbl)
                        n509 = Divide(x=w900, y=w899) -> (x/y=w898:dbl)
                        n510 = Divide(x=w905, y=w904) -> (x/y=w903:dbl)
                        n511 = Round To Nearest(number=w898) -> (nearest integer value=w897:dbl)
                        n512 = Round To Nearest(number=w903) -> (nearest integer value=w902:dbl)
                        n513 = Index Array(array=w909, index (dim 1)=w897, index (dim 2)=w902) -> (element=→"Waveform Graph":i32[])  [unwired: 1 in]
                        n514 = Index Array(array=w909, index (dim 2)=w902) -> (element=w908:i32[][])  [unwired: 2 in]
                        n515 = Transpose 2D Array(2D array=w908) -> (transposed array=w907:i32[][])
                        n516 = local write "Left Graph"(w907) -> ()
                      }
                      event Timeout {
                        n517 = event-data() -> ()  [unwired: 1 in, 3 out]
                        n518 = local read "X"() -> (w943:dbl)
                        n519 = local read "Y"() -> (w942:dbl)
                      }
                    }
                    n520 = Divide(x=w820, y=-1.5446) -> (x/y=w818:dbl)
                    n521 = Round To Nearest(number=w818) -> (nearest integer value=w816:dbl)
                    n522 = Array Size(array=w838) -> (size(s)=w840:i32[])
                    n523 = Less?(x="Bandwidth", y=w816) -> (x < y?=w835:bool)
                    n524 = Not Equal?(x="Bandwidth", y=0.0) -> (x != y?=w834:bool)
                    n525 = Index Array(array=w840, index=2) -> (element=w837:i32)
                    n526 = Index Array(array=w840, index=1) -> (element=w836:i32)
                    n527 = And(x=w835, y=w834) -> (x .and. y?=w833:bool)
                    n528 = Multiply(x=2.0, y="Bandwidth") -> (x*y=w842:dbl)
                    n529 = Index Array(array=w838, index (dim 0)=w816) -> (element=w847:i32[][])  [unwired: 2 in]
                    n530 = event shown="[1] \"Bandwidth\", \"Wavelength\": Value Change" {
                      selector: _ -> [_ _]
                      dyn-events: _ -> [_ _]
                      timeout: 10 -> [_ _]
                      tunnel: [w864 w872] -> w846
                      tunnel: w847 -> [_ _]
                      tunnel: w816 -> [_ w871]
                      tunnel: "Bandwidth" -> [_ w870]
                      tunnel: w838 -> [_ w869]
                      tunnel: w842 -> [_ w868]
                      tunnel: w837 -> [_ w867]
                      tunnel: w836 -> [_ w866]
                      tunnel: w833 -> [_ w865]
                      event Timeout {
                        n531 = event-data() -> ()  [unwired: 1 in, 3 out]
                        n532 = local read "Right Graph"() -> (w864:i32[][])
                      }
                      event "Bandwidth", "Wavelength": Value Change {
                        n533 = event-data() -> ()  [unwired: 1 in, 6 out]
                        n534 = case shown="True" w865 {
                          tunnel: w871 -> [w875 w884]
                          tunnel: w869 -> [w874 w885]
                          tunnel: w868 -> [_ w876]
                          tunnel: [w873 w883] -> w872
                          tunnel: w870 -> [_ w882]
                          tunnel: w867 -> [_ w879]
                          tunnel: w866 -> [_ w878]
                          frame False {
                            n535 = Index Array(array=w874, index (dim 0)=w875) -> (element=w873:i32[][])  [unwired: 2 in]
                          }
                          frame True {
                            n536 = Initialize Array(0 ("element"), w878, w879) -> (w880:i32[][])
                            n537 = for {
                              N: w876 -> [_]
                              tunnel: w885 -> [w894]
                              shift-right: [w892] -> w877
                              shift-left: w880 -> [w889]
                              tunnel: w884 -> [w888]
                              tunnel: w882 -> [w887]
                              i -> [w893]
                              n538 = Subtract(x=w888, y=w887) -> (x-y=w886:dbl)
                              n539 = Add(x=w893, y=w886) -> (x+y=w891:dbl)
                              n540 = Index Array(array=w894, index (dim 0)=w891) -> (element=w890:i32[][])  [unwired: 2 in]
                              n541 = Add ("Add.vi")(x=w890, y=w889) -> (x+y=w892:i32[][])
                            }
                            n542 = Divide(x=w877, y=w876) -> (x/y=w883:dbl[][])
                          }
                        }
                      }
                    }
                    n543 = Round To Nearest(number=w825) -> (nearest integer value=→"X":dbl)
                    n544 = Round To Nearest(number=w824) -> (nearest integer value=→"Y":dbl)
                    n545 = local write "Right Graph"(w846) -> ()
                    n546 = Or(x="Scan again", y="Shut Down") -> (x .or. y?=w832:bool)
                    n547 = event shown="[0] \"Save File\": Value Change" {
                      selector: _ -> [_ _]
                      dyn-events: _ -> [_ _]
                      timeout: 10 -> [_ _]
                      tunnel: w830 -> [w851 _]
                      tunnel: w829 -> [w850 _]
                      event "Save File": Value Change {
                        n548 = event-data() -> ()  [unwired: 1 in, 6 out]
                        n549 = local read "Save File"() -> (w849:bool)
                        n550 = case shown="True" w849 {
                          tunnel: w851 -> [_ w853]
                          tunnel: w850 -> [_ w852]
                          frame False {
                          }
                          frame True {
                            n551 = in-place {
                              in-place-border: w852 -> [w863]
                              in-place-border: w853 -> [w859]
                              n552 = local read "Exposure Time (s)"() -> (w862:sgl)
                              n553 = Path To String(path="path") -> (string=w858:string)
                              n554 = Concatenate Strings(w858, ".tiff" ("string")) -> (w857:string)
                              n555 = String To Path(string=w857) -> (path=w856:path)
                              n556 = Multiply(x=w862, y=sgl 1000.0) -> (x*y=w861:sgl)
                              n557 = call "saveToTIFF.vi"("x array"=w859, "Array"=w863, "selected path"=w856, "SPEC.CCD.Exposure(ms )"=w861) -> ()  [unwired: 7 in]
                            }
                          }
                        }
                      }
                      event Timeout {
                        n558 = event-data() -> ()  [unwired: 1 in, 3 out]
                      }
                    }
                  }
                }
              }
              frame #2 {
                w945 = FALSE ("Visible")
                w944 = T11."Enabled" ("Disabled")
                w946 = T11."Disabled and Grayed Out" ("Disabled")
                n559 = property on="go right Button" class="Bool"("DisabledEnum"=w944) -> ()  [unwired: 2 in, 2 out]
                n560 = property on="Set Temp." class="DigNum (strict)"("DisabledEnum"=w944) -> ()  [unwired: 2 in, 2 out]
                n561 = property on="X" class="DigNum (strict)"("Visible"=w945) -> ()  [unwired: 2 in, 2 out]
                n562 = property on="Scan Step (um)" class="DigNum (strict)"("DisabledEnum"=w944) -> ()  [unwired: 2 in, 2 out]
                n563 = property on="Y" class="DigNum (strict)"("Visible"=w945) -> ()  [unwired: 2 in, 2 out]
                n564 = property on="go left Button" class="Bool"("DisabledEnum"=w944) -> ()  [unwired: 2 in, 2 out]
                n565 = property on="Shutter Control" class="Enum (strict)"("DisabledEnum"=w944) -> ()  [unwired: 2 in, 2 out]
                n566 = property on="Exposure Time (s)" class="DigNum (strict)"("DisabledEnum"=w944) -> ()  [unwired: 2 in, 2 out]
                n567 = property on="VSS (s)" class="Ring (strict)"("DisabledEnum"=w944) -> ()  [unwired: 2 in, 2 out]
                n568 = property on="Scan Start" class="Bool"("DisabledEnum"=w944) -> ()  [unwired: 2 in, 2 out]
                n569 = invoke on="Right Graph" class="IntGraph (strict)" method="Reinit To Default"() -> ()  [unwired: 3 in, 3 out]
                n570 = invoke on="Waveform Graph" class="WFGraph (strict)" method="Reinit To Default"() -> ()  [unwired: 3 in, 3 out]
                n571 = property on="Live View" class="Bool (strict)"("DisabledEnum"=w944) -> ()  [unwired: 2 in, 2 out]
                n572 = property on="Take shot" class="Bool (strict)"("DisabledEnum"=w944) -> ()  [unwired: 2 in, 2 out]
                n573 = property on="HSS (MHz)" class="Ring (strict)"("DisabledEnum"=w944) -> ()  [unwired: 2 in, 2 out]
                n574 = property on="Scan Length (mm)" class="DigNum (strict)"("DisabledEnum"=w944) -> ()  [unwired: 2 in, 2 out]
                n575 = property on="Go back after scan" class="Bool (strict)"("DisabledEnum"=w944) -> ()  [unwired: 2 in, 2 out]
                n576 = property on="Step length (um)" class="DigNum (strict)"("DisabledEnum"=w944) -> ()  [unwired: 2 in, 2 out]
                n577 = invoke on="Left Graph" class="IntGraph (strict)" method="Reinit To Default"() -> ()  [unwired: 3 in, 3 out]
                n578 = property on="path" class="Path"("DisabledEnum"=w946) -> ()  [unwired: 2 in, 2 out]
                n579 = property on="Scan again" class="Bool"("DisabledEnum"=w946) -> ()  [unwired: 2 in, 2 out]
                n580 = property on="Bandwidth" class="DigNum (strict)"("DisabledEnum"=w946) -> ()  [unwired: 2 in, 2 out]
                n581 = property on="Wavelength" class="Slide (strict)"("DisabledEnum"=w946) -> ()  [unwired: 2 in, 2 out]
                n582 = property on="Waveform Graph" class="WFGraph (strict)"("DisabledEnum"=w946) -> ()  [unwired: 2 in, 2 out]
                n583 = property on="Save File" class="Bool (strict)"("DisabledEnum"=w946) -> ()  [unwired: 2 in, 2 out]
              }
            }
          }
        }
      }
    }
    frame #3 {
      n584 = flat-sequence {
        frame #0 {
          n585 = in-place {
            n586 = call <userlib>:"CoolerOFF.vi"() -> ("error out"=w948:errorcluster)  [unwired: 2 in, 1 out]
            n587 = call <userlib>:"SetShutter.vi"("type"=Shutter_type_typedef."TTL Low", "mode"=Shutter_mode_typedef."Close", "error in (no error)"=w948) -> ()  [unwired: 11 in, 2 out]
            n588 = while {
              stop <- w952 stop-if-true
              n589 = flat-sequence {
                tunnel: [w955] -> w952
                frame #0 {
                  n590 = call <userlib>:"GetTemperature.vi"() -> ("status"=w953:T1, "temperature"=w954:i32)  [unwired: 4 in, 2 out]
                  n591 = local write "Temp"(w954) -> ()
                  n592 = local write "temp. status 2"(w953) -> ()
                  n593 = Greater Or Equal?(x=w954, y=0) -> (x >= y?=w955:bool)
                }
                frame #1 {
                  n594 = Wait (ms)(milliseconds to wait=u32 2000) -> ()  [unwired: 1 out]
                }
              }
              n595 = Not(x=w952) -> (.not. x?=→"recovering temperature":bool)
            }
          }
        }
        frame #1 {
          n596 = in-place {
            n597 = call <userlib>:"AbortAcquisition.vi"() -> ("error out"=w959:errorcluster)  [unwired: 2 in, 1 out]
            n598 = call <userlib>:"ShutDown.vi"("error in (no error)"=w959) -> ()  [unwired: 1 in, 2 out]
          }
          n599 = control-ref of="This VI"() -> (w958:refnum<vi>)
          n600 = invoke class="VI" method="Default Vals.Reinit All"(reference=w958) -> ()  [unwired: 2 in, 3 out]
          n601 = invoke on="Shut Down" class="Bool (strict)" method="Reinit To Default"() -> ()  [unwired: 3 in, 3 out]
        }
      }
    }
  }
